vi "Test - All-In-One - SLAM Configuration -DISP B (SubVI).vi"(0 "START TEST":bool, 1 "STOP TEST":bool, 2 "NEXT STEP":bool, 3 "HOLD STEP":bool, 4 "Test Folder":path, 5 "Error Input":errorcluster, 7 "SLAM Test Cluster":T1={"Load Test"=0, "New Test Name"="", "Test Description"="", "Step Select"=0, "Save Test"=FALSE, "Erase Test"=FALSE, "Max Steps"=15, "Loop Limit"=5, "Continue at Loop Limit?"=FALSE, "Step N"=2, "Test Array (Standard)"=[{"Step Number"=0, "Step Description"="Turn ON H2O VLV", "Step Time Target"=1.0, "Step Time Unit"=0, "Step End Action"=0}, {"Step Number"=1, "Step Description"="H2O OFF, Soap ON", "Step Time Target"=1.0, "Step Time Unit"=0, "Step End Action"=0}, {"Step Number"=2, "Step Description"="Scrub Delay Time", "Step Time Target"=4.0, "Step Time Unit"=0, "Step End Action"=0}, {"Step Number"=3, "Step Description"="Rinse Time", "Step Time Target"=20.0, "Step Time Unit"=0, "Step End Action"=0}, {"Step Number"=4, "Step Description"="Signal Complete", "Step Time Target"=1.0, "Step Time Unit"=0, "Step End Action"=0}, {"Step Number"=5, "Step Description"="Re-Initialize", "Step Time Target"=0.5, "Step Time Unit"=0, "Step End Action"=3}], "Test Array (Custom)"=[{"Digital Outputs"=[TRUE, TRUE, FALSE, FALSE, FALSE, FALSE, FALSE, FALSE]}, {"Digital Outputs"=[FALSE, TRUE, TRUE, FALSE, FALSE, FALSE, FALSE, FALSE]}, {"Digital Outputs"=[FALSE, FALSE, FALSE, TRUE, FALSE, FALSE, FALSE, FALSE]}, {"Digital Outputs"=[TRUE, FALSE, FALSE, FALSE, TRUE, TRUE, FALSE, FALSE]}, {"Digital Outputs"=[FALSE, FALSE, FALSE, FALSE, FALSE, FALSE, TRUE, FALSE]}, {"Digital Outputs"=[FALSE, FALSE, FALSE, FALSE, FALSE, FALSE, FALSE, FALSE]}]} {"Test Array (Standard)"."Step End Action" items=["Go to Next Step", "Loop to Step 0", "Loop to Step N", "Stop Test Mode", "Stop Program"]; "Test Array (Standard)"."Step Time Unit" items=["sec", "min", "hr"]; "Test Array (Standard)"."Step Time Target" min=0.001 format="%#.3f"; "Test Array (Standard)"."Step Number" min=0 step=1; "Load Test" items=["123", "a", "b", "c"]; "Step Select" step=1}, 9 "SLAM Test Cluster Ref":refnum<vi>) -> (11 "Stop Program?":bool, 13 "Test Running?":bool, 14 "Test Display":string="Mode: OFF  (Press Start to Begin)\r\r\r    ", 15 "Test Output":cluster{"Digital Outputs":bool[]}, 16 "Step Complete?":bool=TRUE, 17 "Step Number":u16, 18 "Loop Number":u16, 19 "Error Output":errorcluster)   [LabVIEW 2012]
panel:
  # "Extra (Unused)"
  # "Red LED's"
  # "Rinse Green LED"
  # "+1 on Hand Remove"
  # "Scrub Green LED"
  # "Soap Control"
  # "Water Green LED"
  # "H2O Control"
  # "Scroll"
  # "Step"
  # "Description"
  # "Time Target"
  # "End Action"
  # "Total #\nof Steps"
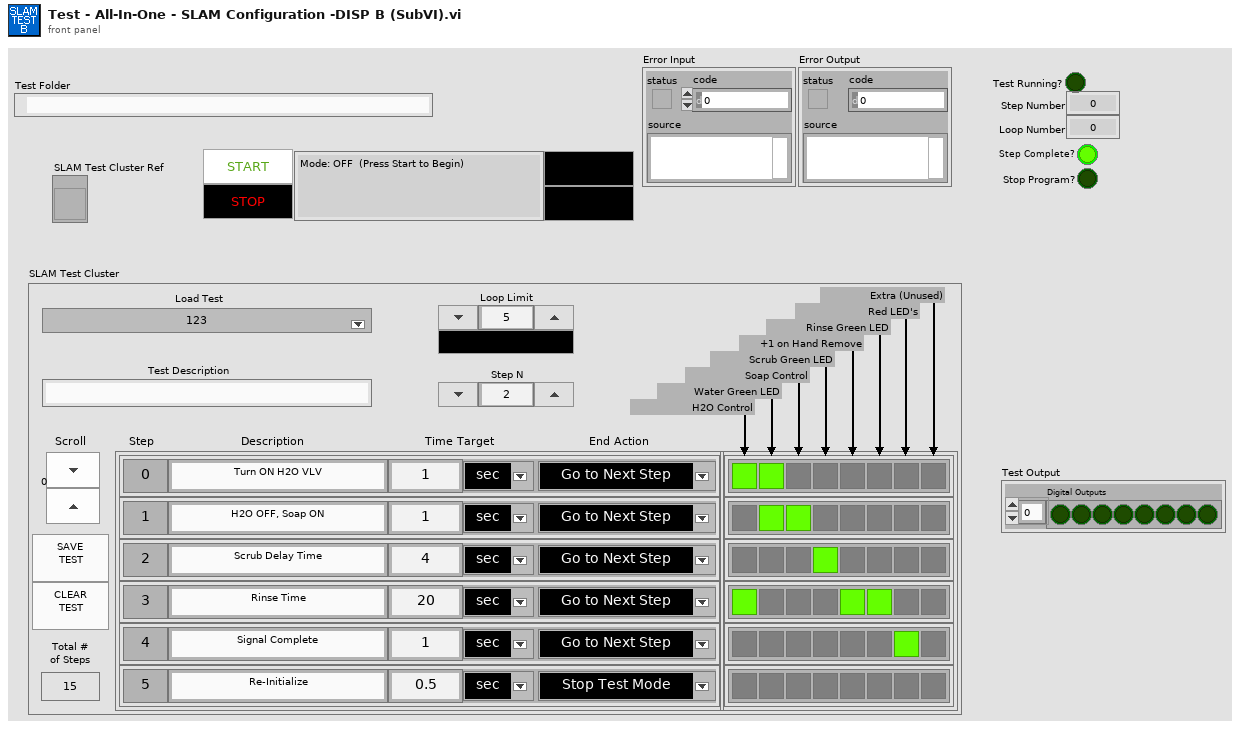
[diagram p1: front panel]
types:
  T1 = cluster{"Load Test":u16, "New Test Name":string, "Test Description":string, "Step Select":u16, "Save Test":bool, "Erase Test":bool, "Max Steps":u16, "Loop Limit":u16, "Continue at Loop Limit?":bool, "Step N":u16, "Test Array (Standard)":cluster{"Step Number":i32, "Step Description":string, "Step Time Target":dbl, "Step Time Unit":u16, "Step End Action":u16}[], "Test Array (Custom)":cluster{"Digital Outputs":bool[]}[]}
  T2 = cluster{"Load Test Ring":i32, "New Test Name":i32, "Test Description":i32, "Step Select":i32, "Save Test":i32, "Erase Test":i32, "Max Steps":i32, "Loop Limit":i32, "Continue at Loop Limit":i32, "Step N":i32, "Test Array (Standard)":i32, "Test Array (Custom)":i32}
  T3 = enum8{"Enabled", "Disabled", "Disabled and Grayed Out"}
  T4 = cluster{"Step Number":i32, "Step Description":string, "Step Time Target":dbl, "Step Time Unit":u16, "Step End Action":u16}[]
  T5 = enum16{"open", "replace", "create", "open or create", "replace or create", "replace or create with confirmation"}
  T6 = cluster{"Step Number":i32, "Step Description":string, "Step Time Target":dbl, "Step Time Unit":u16, "Step End Action":u16}
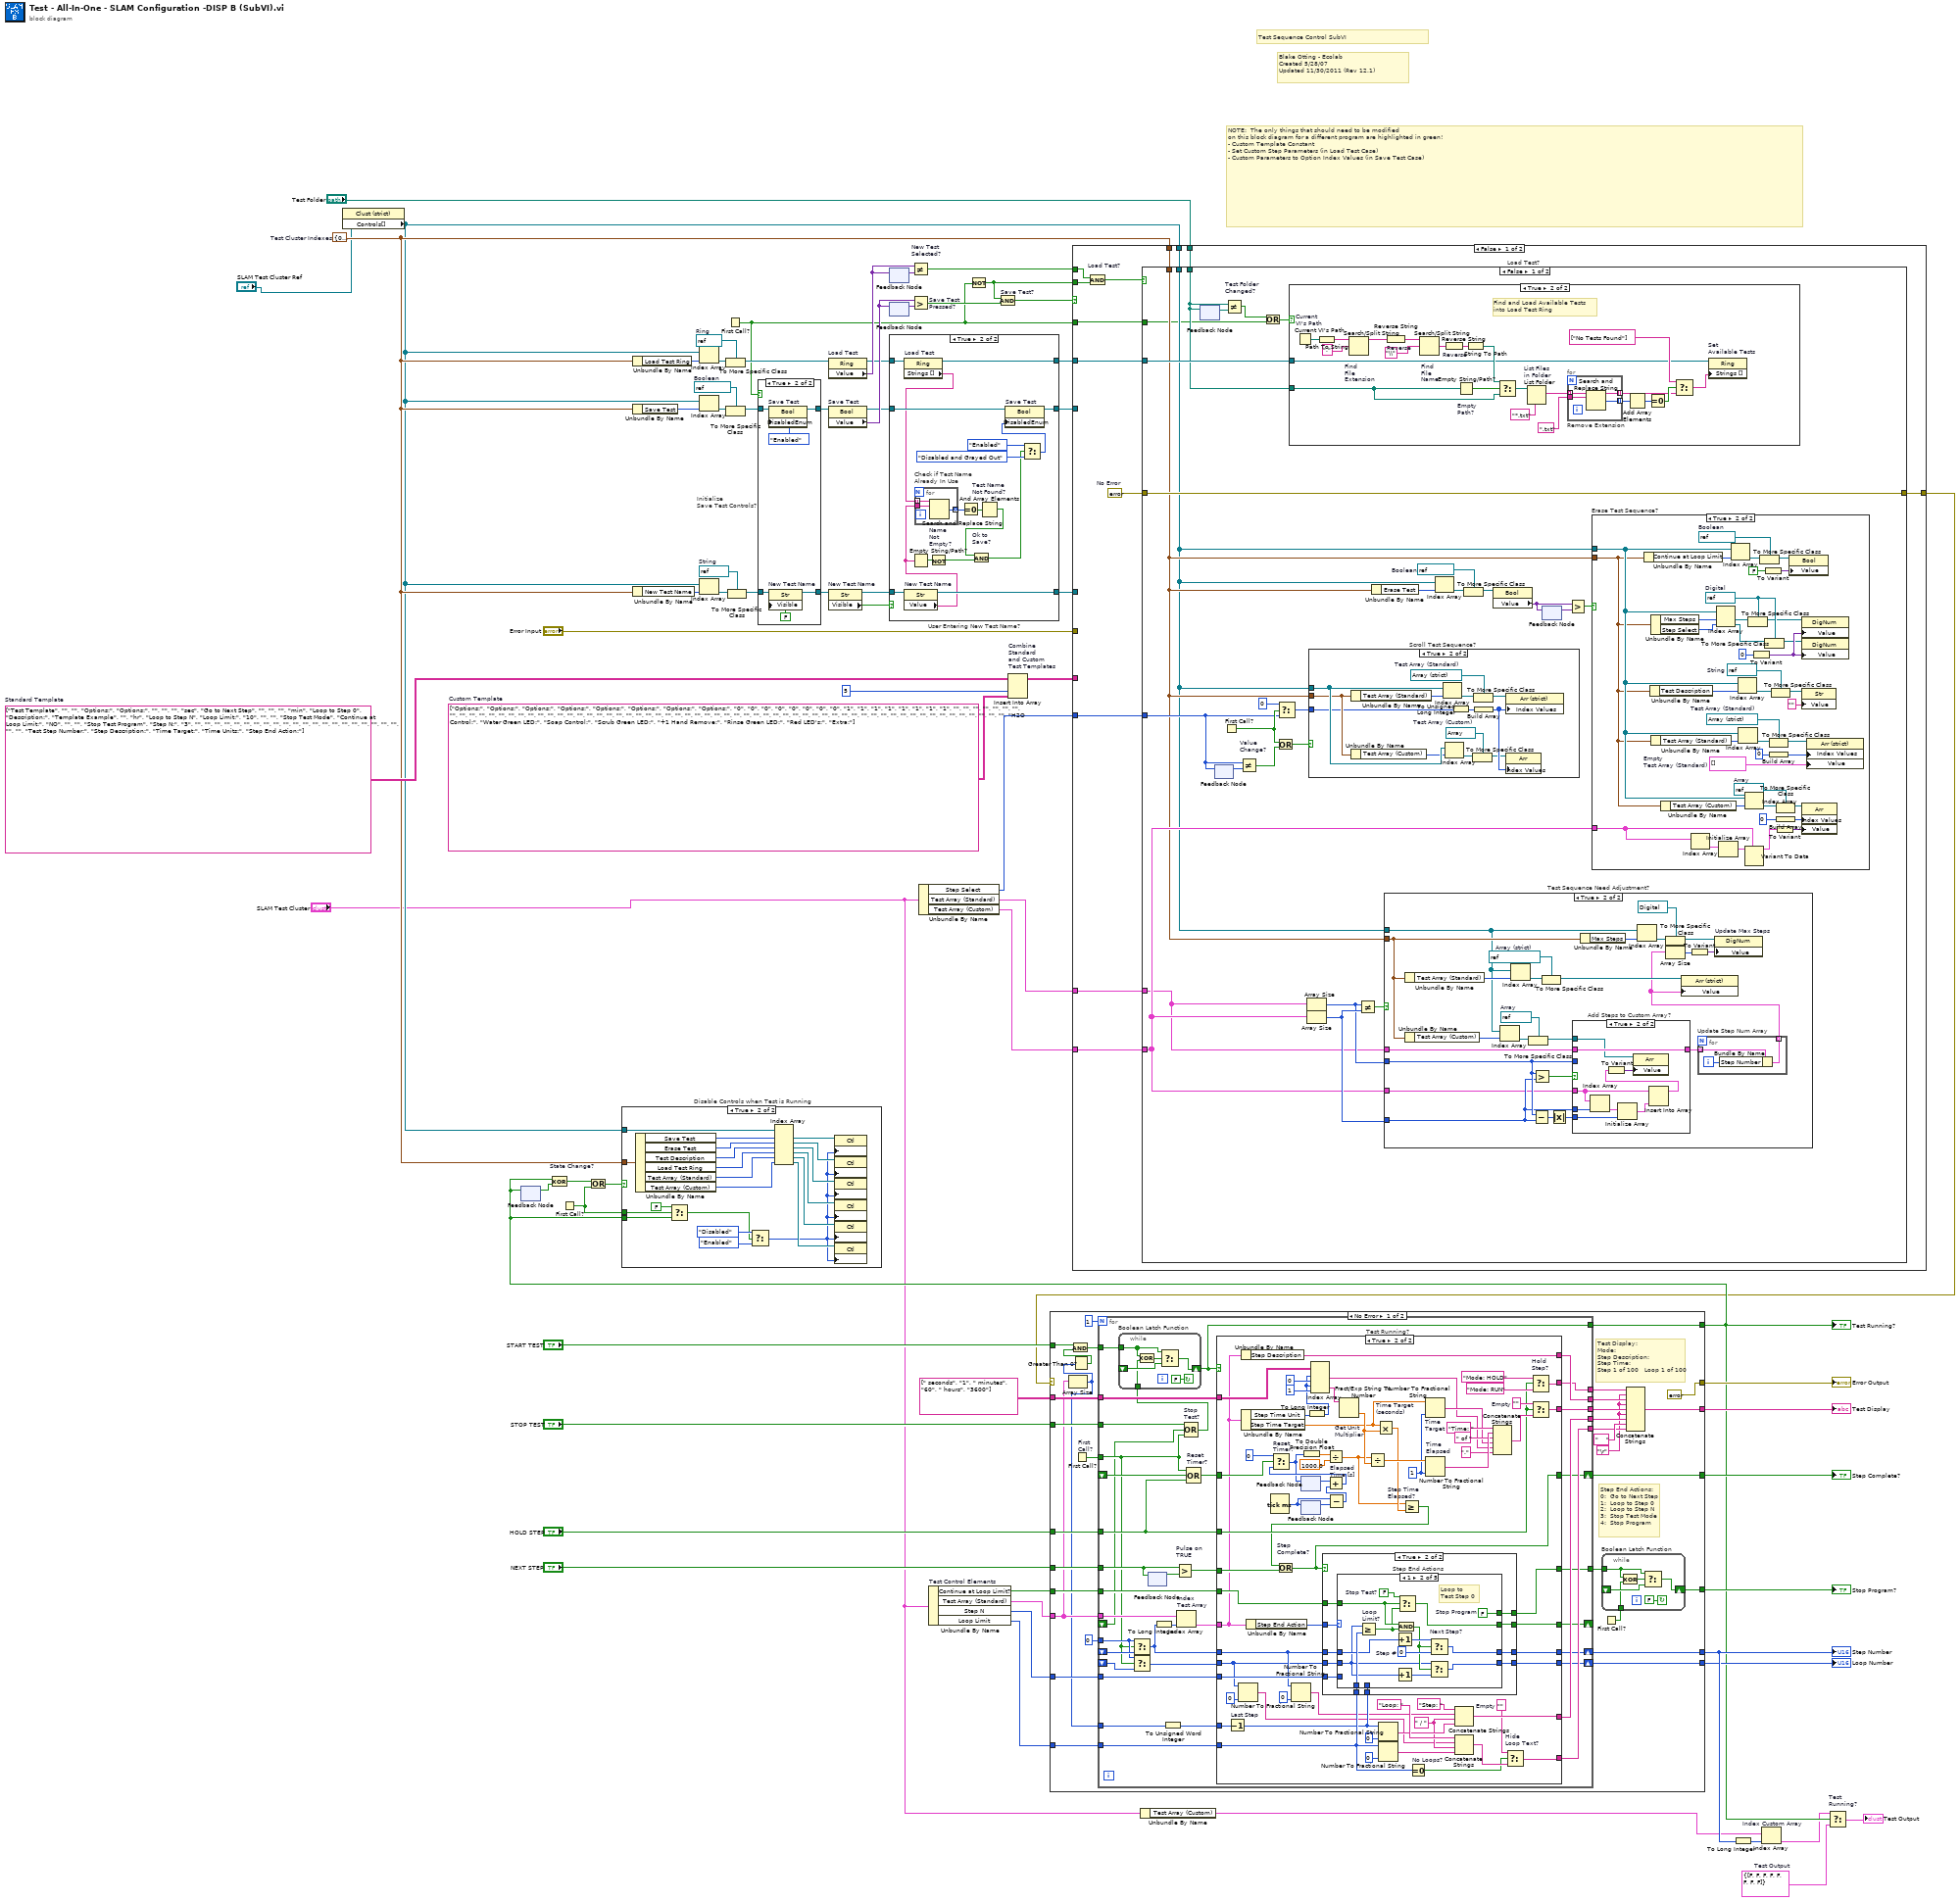
[diagram p0: block diagram]
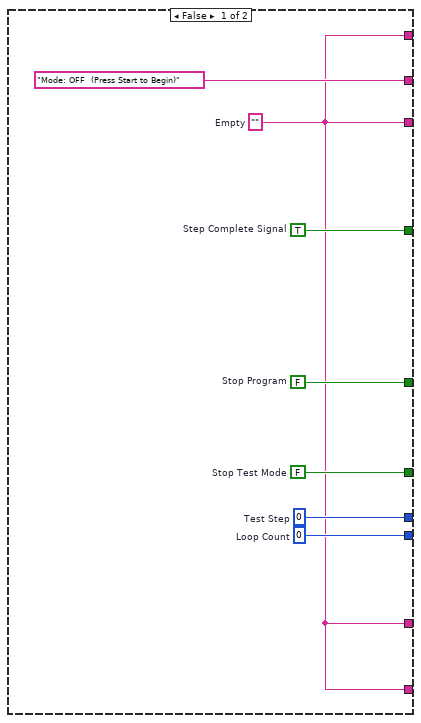
[diagram p3: hidden frame]
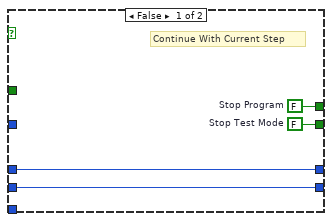
[diagram p4: hidden frame]
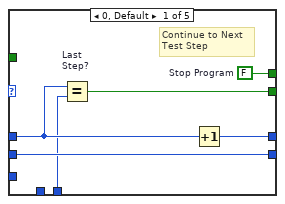
[diagram p5: hidden frame]
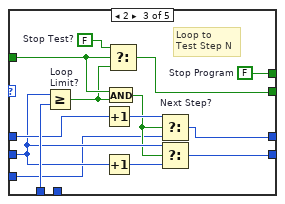
[diagram p6: hidden frame]
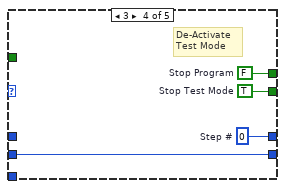
[diagram p7: hidden frame]
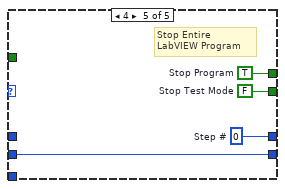
[diagram p8: hidden frame]
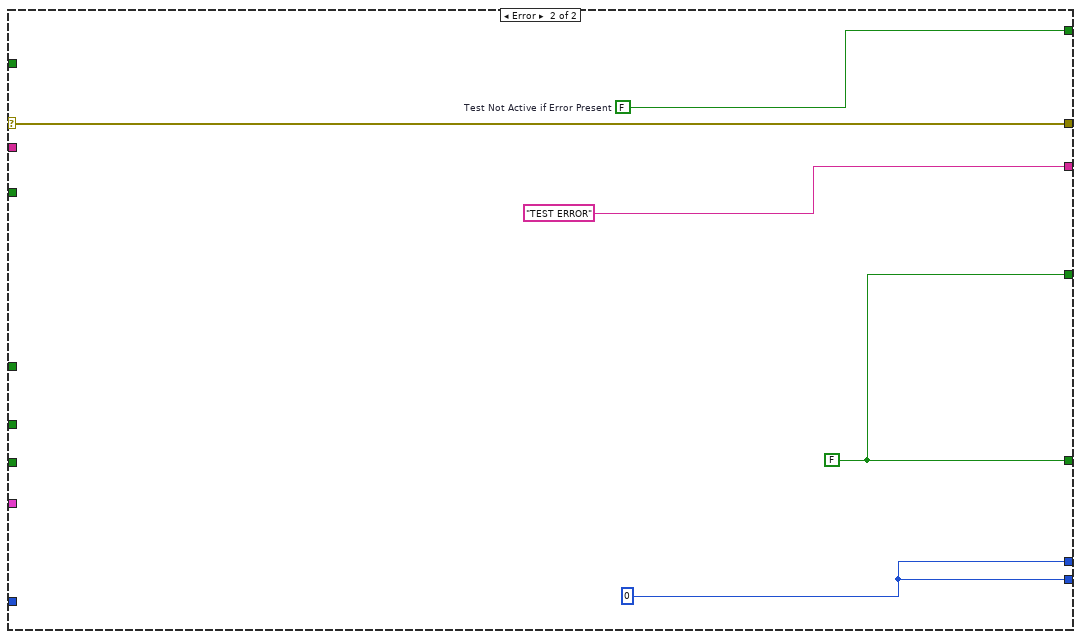
[diagram p9: hidden frame]
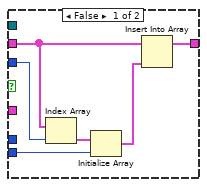
[diagram p13: hidden frame]
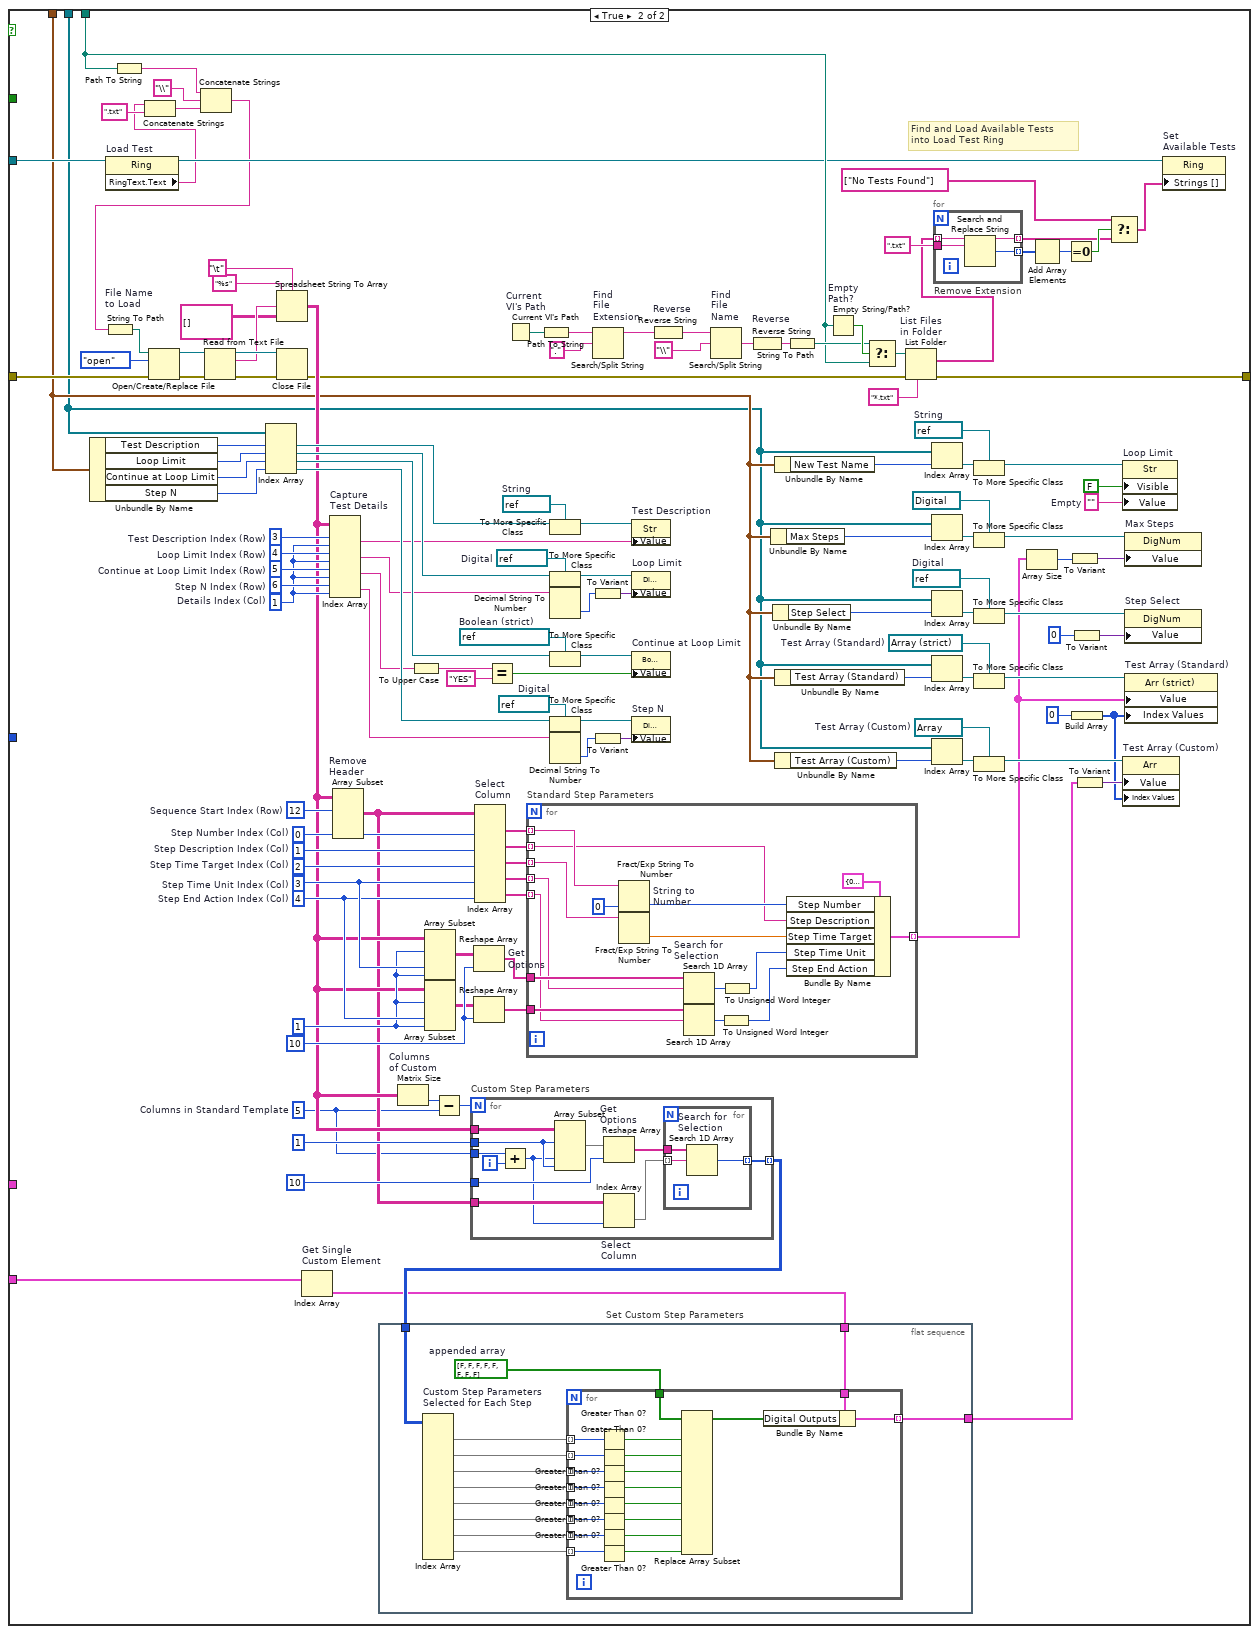
[diagram p17: hidden frame]
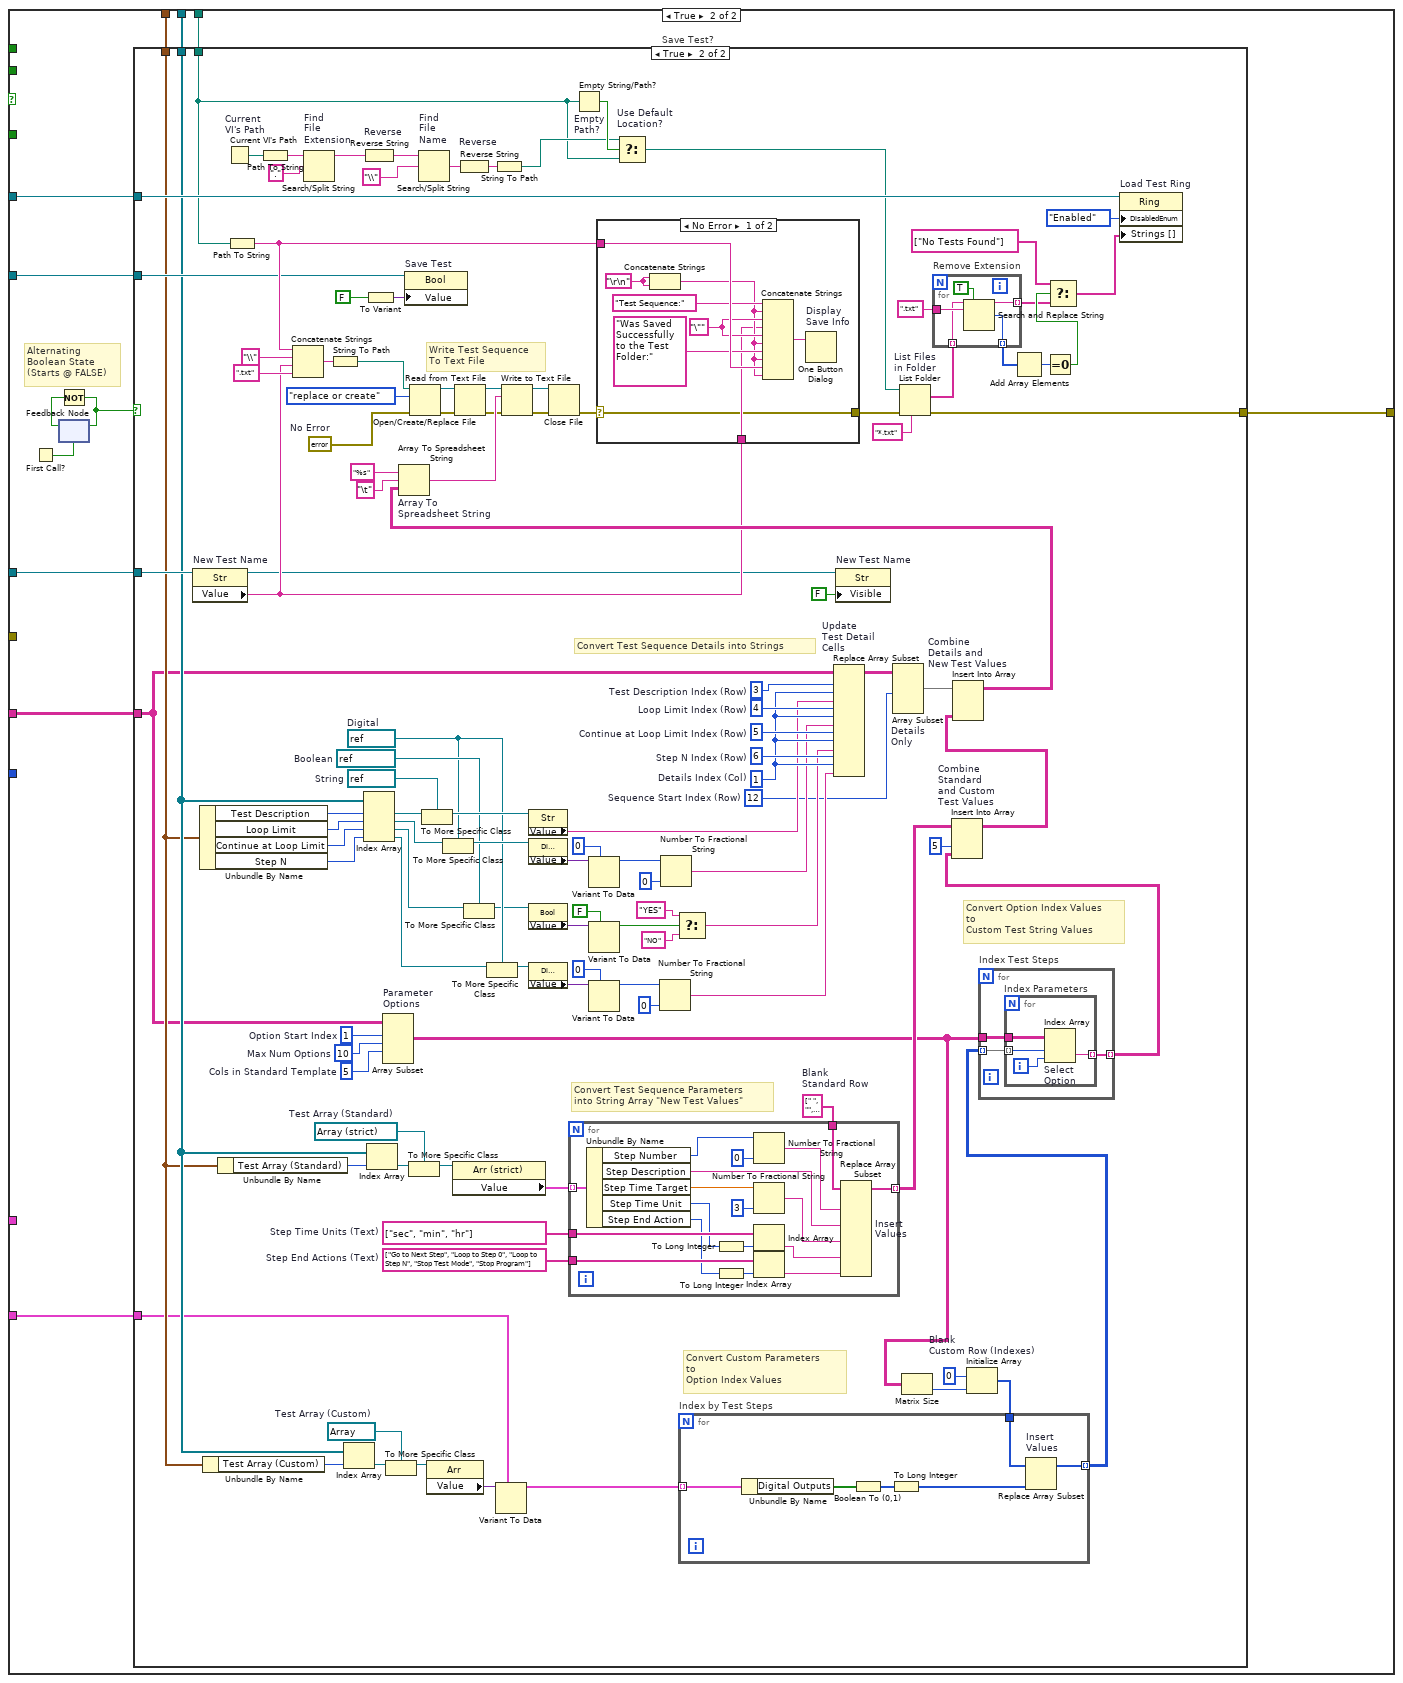
[diagram p18: hidden frame]
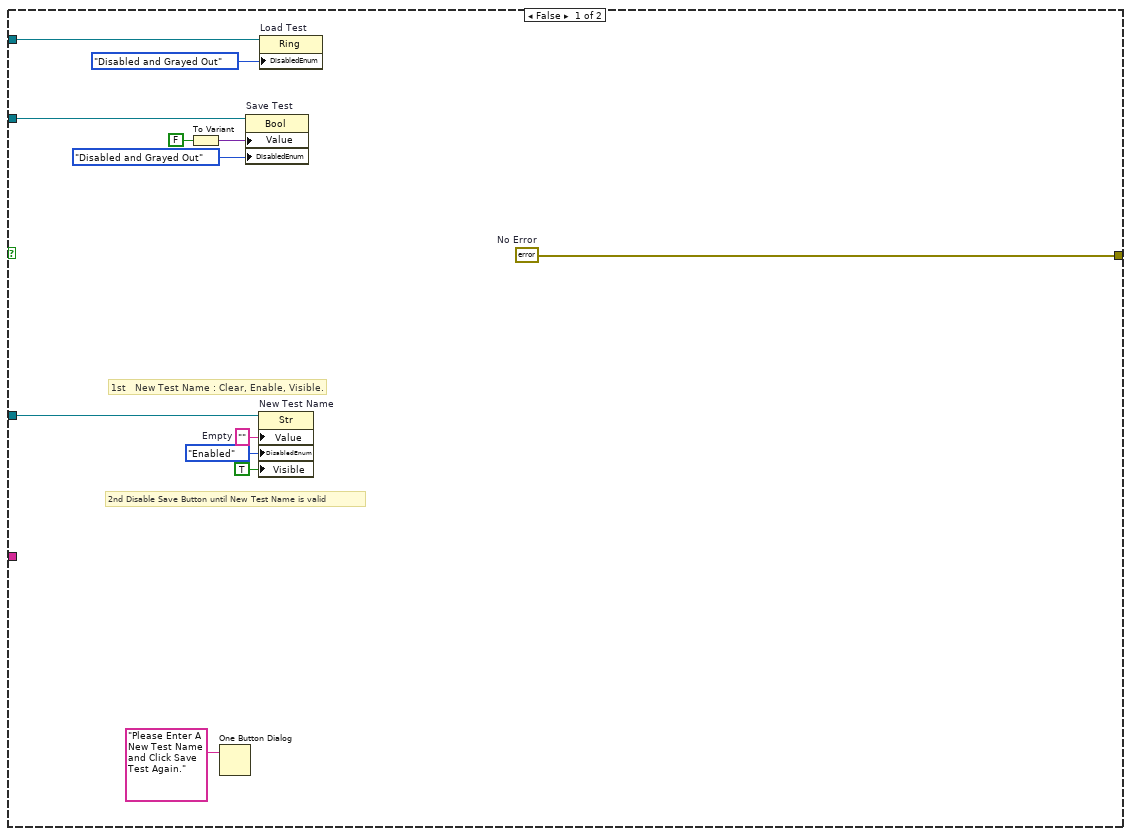
[diagram p19: hidden frame]
diagram:
  w2 = cluster{"Digital Outputs":bool[]} {"Digital Outputs"=[FALSE, FALSE, FALSE, FALSE, FALSE, FALSE, FALSE, FALSE]}  # Test Output
  w31 = refnum<vi> refnum  # Ring
  w53 = refnum<vi> refnum  # Boolean
  w57 = refnum<vi> refnum  # String
  w62 = string[][] [["Options:", "Options:", "Options:", "Options:", "Options:", "Options:", "Options:", "Options:"], ["0", "0", "0", "0", "0", "0", "0", "0"], ["1", "1", "1", "1", "1", "1", "1", "1"], ["", "", "", "", "", "", "", ""], ["", "", "", "", "", "", "", ""], ["", "", "", "", "", "", "", ""], ["", "", "", "", "", "", "", ""], ["", "", "", "", "", "", "", ""], ["", "", "", "", "", "", "", ""], ["", "", "", "", "", "", "", ""], ["", "", "", "", "", "", "", ""], ["H2O Control:", "Water Green LED:", "Soap Control:", "Scrub Green LED:", "+1 Hand Remove:", "Rinse Green LED:", "Red LED's:", "Extra:"]]  # Custom Template
  w64 = T2 {"Load Test Ring"=0, "New Test Name"=1, "Test Description"=2, "Step Select"=3, "Save Test"=4, "Erase Test"=5, "Max Steps"=6, "Loop Limit"=7, "Continue at Loop Limit"=8, "Step N"=9, "Test Array (Standard)"=10, "Test Array (Custom)"=11}  # Test Cluster Indexes
  w69 = string[][] [["Test Template", "", "", "Options:", "Options:"], ["", "", "", "sec", "Go to Next Step"], ["", "", "", "min", "Loop to Step 0"], ["Description:", "Template Example", "", "hr", "Loop to Step N"], ["Loop Limit:", "10", "", "", "Stop Test Mode"], ["Continue at Loop Limit:", "NO", "", "", "Stop Test Program"], ["Step N:", "3", "", "", ""], ["", "", "", "", ""], ["", "", "", "", ""], ["", "", "", "", ""], ["", "", "", "", ""], ["Test Step Number:", "Step Description:", "Time Target:", "Time Units:", "Step End Action:"]]  # Standard Template
  # "NOTE:  The only things that should need to be modified\non this block diagram for a different program are highlighted in green!\n- Custom Template Constant\n- Set Custom Step Parameters (in Load Test Case)\n- Custom Parameters to Option Index Values (in Save Test Case)"
  # "Blake Otting - Ecolab\nCreated 5/28/07\nUpdated 11/30/2011 (Rev 12.1)"
  # "Test Sequence Control SubVI"
  n1 = property class="Clust (strict)"(reference="SLAM Test Cluster Ref") -> ("Controls[]"=w63:refnum<vi>[])  [unwired: 1 in, 2 out]
  n2 = feedback #1() -> (w28:bool)  [unwired: 1 in]
  n3 = First Call?() -> (First Call?: T/F=w25:bool)
  n4 = Unbundle By Name(w64) -> ("Load Test Ring"=w32:i32)
  n5 = Unbundle By Name(w64) -> ("Save Test"=w55:i32)
  n6 = Unbundle By Name(w64) -> ("New Test Name"=w59:i32)
  n7 = Index Array(array=w63, index=w32) -> (element=w30:refnum<vi>)
  n8 = Index Array(array=w63, index=w55) -> (element=w54:refnum<vi>)
  n9 = Index Array(array=w63, index=w59) -> (element=w58:refnum<vi>)
  n10 = First Call?() -> (First Call?: T/F=w11:bool)
  n11 = To More Specific Class(target class=w31, reference=w30) -> (specific class reference=w29:refnum<vi>)  [unwired: 1 in, 1 out]
  n12 = To More Specific Class(target class=w53, reference=w54) -> (specific class reference=w42:refnum<vi>)  [unwired: 1 in, 1 out]
  n13 = To More Specific Class(target class=w57, reference=w58) -> (specific class reference=w44:refnum<vi>)  [unwired: 1 in, 1 out]
  n14 = case "Initialize\nSave Test Controls?" shown="True" w11 {
    tunnel: w42 -> [w70 w77]
    tunnel: [w70 w76] -> w41
    tunnel: w44 -> [w71 w75]
    tunnel: [w71 w74] -> w43
    frame False {
    }
    frame True {
      n15 = property on="Save Test" class="Bool"(reference=w77, "DisabledEnum"=T3."Enabled" ("Disabled")) -> (reference out=w76:refnum<vi>)  [unwired: 1 in, 1 out]
      n16 = property on="New Test Name" class="Str"(reference=w75, "Visible"=FALSE) -> (reference out=w74:refnum<vi>)  [unwired: 1 in, 1 out]
    }
  }
  n17 = property on="Load Test" class="Ring"(reference=w29) -> (reference out=w37:refnum<vi>, "Value"=w38:variant)  [unwired: 1 in, 1 out]
  n18 = property on="Save Test" class="Bool"(reference=w41) -> (reference out=w47:refnum<vi>, "Value"=w51:variant)  [unwired: 1 in, 1 out]
  n19 = property on="New Test Name" class="Str"(reference=w43) -> (reference out=w49:refnum<vi>, "Visible"=w50:bool)  [unwired: 1 in, 1 out]
  n20 = case "User Entering New Test Name?" shown="True" w50 {
    tunnel: w49 -> [w80 w93]
    tunnel: w37 -> [w79 w92]
    tunnel: [w80 w88] -> w46
    tunnel: [w79 w87] -> w48
    tunnel: w47 -> [w78 w86]
    tunnel: [w78 w85] -> w45
    frame False {
    }
    frame True {
      n21 = property on="Load Test" class="Ring"(reference=w92) -> (reference out=w87:refnum<vi>, "Strings []"=w82:string[])  [unwired: 1 in, 1 out]
      n22 = property on="New Test Name" class="Str"(reference=w93) -> (reference out=w88:refnum<vi>, "Value"=w81:string)  [unwired: 1 in, 1 out]
      n23 = Empty String/Path?(string/path=w81) -> (empty?=w94:bool)
      n24 = for "Check if Test Name\nAlready In Use" {
        tunnel: w82 -> [w100] mode=indexing
        tunnel: w81 -> [w99]
        tunnel: [w98] -> w97 mode=indexing
        n25 = Search and Replace String(input string=w100, search string=w99) -> (number of replacements=w98:i32)  [unwired: 6 in, 3 out]
      }
      n26 = Not "Name\nNot\nEmpty?"(x=w94) -> (.not. x?=w89:bool)
      n27 = Equal To 0?(x=w97) -> (x = 0?=w96:bool[])
      n28 = And Array Elements "Test Name\nNot Found?"(Boolean array=w96) -> (logical AND=w95:bool)
      n29 = And "Ok to\nSave?"(x=w95, y=w89) -> (x .and. y?=w83:bool)
      n30 = Select(t=T3."Enabled" ("Disabled"), s=w83, f=T3."Disabled and Grayed Out" ("Disabled")) -> (s? t:f=w84:T3)
      n31 = property on="Save Test" class="Bool"(reference=w86, "DisabledEnum"=w84) -> (reference out=w85:refnum<vi>)  [unwired: 1 in, 1 out]
    }
  }
  n32 = feedback #2() -> (w39:variant)  [unwired: 1 in]
  n33 = feedback-in #2(w38) -> ()
  n34 = feedback #3() -> (w52:variant)  [unwired: 1 in]
  n35 = feedback-in #3(w51) -> ()
  n36 = Not Equal? "New Test\nSelected?"(x=w38, y=w39) -> (x != y?=w7:bool)
  n37 = Greater? "Save Test\nPressed?"(x=w51, y=w52) -> (0:w36:bool)
  n38 = Unbundle By Name("SLAM Test Cluster") -> ("Step Select"=w19:u16, "Test Array (Standard)"=w21:T4, "Test Array (Custom)"=w20:cluster{"Digital Outputs":bool[]}[])
  n39 = Unbundle By Name "Test Control Elements"("SLAM Test Cluster") -> ("Continue at Loop Limit?"=w24:bool, "Test Array (Standard)"=w9:T4, "Step N"=w23:u16, "Loop Limit"=w22:u16)
  n40 = Not(x=w11) -> (.not. x?=w35:bool)
  n41 = And "Save Test?"(x=w35, y=w36) -> (x .and. y?=w40:bool)
  n42 = Insert Into Array "Combine\nStandard\nand Custom\nTest Templates"(array=w69, index (col)=5 ("disabled index (col)"), new element=w62) -> (w56:string[][])  [unwired: 1 in]
  n43 = case shown="False" w40 {
    tunnel: "Test Folder" -> [w109 w465]
    tunnel: w20 -> [w110 w466]
    tunnel: w56 -> [_ w467]
    tunnel: w64 -> [w112 w471]
    tunnel: w63 -> [w113 w472]
    tunnel: w45 -> [_ w470]
    tunnel: w46 -> [_ w469]
    tunnel: w48 -> [w111 w468]
    tunnel: [w104 w464] -> w10
    tunnel: "Error Input" -> [_ _]
    tunnel: w7 -> [w106 _]
    tunnel: w11 -> [w108 _]
    tunnel: w35 -> [w105 _]
    tunnel: w19 -> [w103 _]
    tunnel: w21 -> [w102 _]
    frame False {
      w101 = errorcluster {"status"=FALSE, "code"=0, "source"=""}  # No Error
      n44 = And "Load Test?"(x=w106, y=w105) -> (x .and. y?=w107:bool)
      n45 = case "Load Test?" shown="False" w107 {
        tunnel: w113 -> [w120 w265]
        tunnel: w112 -> [w121 w266]
        tunnel: w110 -> [w122 w397]
        tunnel: [w141 w274] -> w104
        tunnel: w101 -> [w141 w267]
        tunnel: w111 -> [w140 w271]
        tunnel: w108 -> [w115 _]
        tunnel: w109 -> [w117 w272]
        tunnel: w103 -> [w133 _]
        tunnel: w102 -> [w119 _]
        frame False {
          w128 = refnum<vi> refnum  # Boolean
          n46 = feedback #4() -> (w118:path)  [unwired: 1 in]
          n47 = feedback-in #4(w117) -> ()
          n48 = feedback #5() -> (w134:u16)  [unwired: 1 in]
          n49 = feedback-in #5(w133) -> ()
          n50 = First Call?() -> (First Call?: T/F=w138:bool)
          n51 = Not Equal? "Test Folder\nChanged?"(x=w117, y=w118) -> (x != y?=w116:bool)
          n52 = Not Equal? "Value\nChange?"(x=w133, y=w134) -> (x != y?=w135:bool)
          n53 = Or(x=w116, y=w115) -> (x .or. y?=w114:bool)
          n54 = Or(x=w138, y=w135) -> (x .or. y?=w136:bool)
          n55 = Select(t=u16 0 ("upper limit"), s=w138, f=w133) -> (s? t:f=w139:u16)
          n56 = case shown="True" w114 {
            tunnel: w140 -> [_ w239]
            tunnel: w117 -> [_ w238]
            frame False {
            }
            frame True {
              # "Find and Load Available Tests \ninto Load Test Ring"
              n57 = Current VI's Path "Current\nVI's Path"() -> (path=w249:path)
              n58 = Path To String(path=w249) -> (string=w254:string)
              n59 = Search/Split String "Find\nFile \nExtension"(string=w254, search string/char (-)=".") -> (substring before match=w253:string)  [unwired: 1 in, 2 out]
              n60 = Reverse String "Reverse"(1:w253) -> (0:w252:string)
              n61 = Search/Split String "Find\nFile \nName"(string=w252, search string/char (-)="\\") -> (match + rest of string=w250:string)  [unwired: 1 in, 2 out]
              n62 = Reverse String "Reverse"(1:w250) -> (0:w256:string)
              n63 = Empty String/Path? "Empty\nPath?"(string/path=w238) -> (empty?=w248:bool)
              n64 = String To Path(string=w256) -> (path=w247:path)
              n65 = Select(t=w247, s=w248, f=w238) -> (s? t:f=w257:path)
              n66 = List Folder "List Files\nin Folder"(path=w257, pattern="*.txt") -> (filenames=w259:string[])  [unwired: 1 in, 4 out]
              n67 = for "Remove Extension" {
                tunnel: w259 -> [w262] mode=indexing
                tunnel: ".txt" ("pattern") -> [w263]
                tunnel: [w261] -> w240 mode=indexing
                tunnel: [w260] -> w245 mode=indexing
                n68 = Search and Replace String(input string=w262, search string=w263) -> (result string=w261:string, number of replacements=w260:i32)  [unwired: 6 in, 2 out]
              }
              n69 = Add Array Elements(numeric array=w245) -> (sum=w244:i32)
              n70 = Equal To 0?(x=w244) -> (x = 0?=w243:bool)
              n71 = Select(t=string[] ["No Tests Found"], s=w243, f=w240) -> (s? t:f=w242:string[])
              n72 = property on="Set\nAvailable Tests" class="Ring"(reference=w239, "Strings []"=w242) -> ()  [unwired: 1 in, 2 out]
            }
          }
          n73 = Array Size(array=w119) -> (size(s)=w123:i32)
          n74 = Array Size(array=w122) -> (size(s)=w124:i32)
          n75 = case "Scroll Test Sequence?" shown="True" w136 {
            tunnel: w120 -> [_ w237]
            tunnel: w121 -> [_ w236]
            tunnel: w139 -> [_ w225]
            frame False {
            }
            frame True {
              w235 = refnum<vi> refnum  # Test Array (Custom)
              w232 = refnum<vi> refnum  # Test Array (Standard)
              n76 = Unbundle By Name(w236) -> ("Test Array (Standard)"=w233:i32)
              n77 = Unbundle By Name(w236) -> ("Test Array (Custom)"=w234:i32)
              n78 = Index Array(array=w237, index=w233) -> (element=w226:refnum<vi>)
              n79 = Index Array(array=w237, index=w234) -> (element=w229:refnum<vi>)
              n80 = To Unsigned Long Integer(number=w225) -> (unsigned 32bit integer=w228:u32)
              n81 = To More Specific Class(target class=w235, reference=w229) -> (specific class reference=w230:refnum<vi>)  [unwired: 1 in, 1 out]
              n82 = To More Specific Class(target class=w232, reference=w226) -> (specific class reference=w227:refnum<vi>)  [unwired: 1 in, 1 out]
              n83 = Build Array(w228) -> (w231:u32[])
              n84 = property class="Arr (strict)"(reference=w227, "Index Values"=w231) -> ()  [unwired: 1 in, 2 out]
              n85 = property class="Arr"(reference=w230, "Index Values"=w231) -> ()  [unwired: 1 in, 2 out]
            }
          }
          n86 = Not Equal?(x=w123, y=w124) -> (x != y?=w125:bool)
          n87 = Unbundle By Name(w121) -> ("Erase Test"=w126:i32)
          n88 = case "Test Sequence Need Adjustment?" shown="True" w125 {
            tunnel: w121 -> [_ w150]
            tunnel: w120 -> [_ w149]
            tunnel: w123 -> [_ w148]
            tunnel: w119 -> [_ w147]
            tunnel: w124 -> [_ w146]
            tunnel: w122 -> [_ w145]
            frame False {
            }
            frame True {
              w162 = refnum<vi> refnum  # Array
              w159 = refnum<vi> refnum  # Array (strict)
              n89 = Unbundle By Name(w150) -> ("Test Array (Standard)"=w160:i32)
              n90 = Unbundle By Name(w150) -> ("Test Array (Custom)"=w161:i32)
              n91 = Index Array(array=w149, index=w161) -> (element=w158:refnum<vi>)
              n92 = Index Array(array=w149, index=w160) -> (element=w157:refnum<vi>)
              n93 = To More Specific Class(target class=w162, reference=w158) -> (specific class reference=w144:refnum<vi>)  [unwired: 1 in, 1 out]
              n94 = Subtract(x=w148, y=w146) -> (x-y=w165:i32)
              n95 = Greater?(x=w148, y=w146) -> (0:w164:bool)
              n96 = To More Specific Class(target class=w159, reference=w157) -> (specific class reference=w143:refnum<vi>)  [unwired: 1 in, 1 out]
              n97 = Absolute Value(x=w165) -> (abs(x)=w166:i32)
              n98 = case "Add Steps to Custom Array?" shown="True" w164 {
                tunnel: w144 -> [_ w173]
                tunnel: w146 -> [_ w174]
                tunnel: w145 -> [_ w180]
                tunnel: w147 -> [w168 w175]
                tunnel: w166 -> [w172 w176]
                tunnel: w148 -> [w171 _]
                tunnel: [w167 w175] -> w163
                frame False {
                  n99 = Index Array(array=w168, index=w171) -> (element=w170:T6)
                  n100 = Initialize Array(w170, w172) -> (w169:T4)
                  n101 = Insert Into Array(array=w168, new element=w169) -> (w167:T4)  [unwired: 1 in]
                }
                frame True {
                  n102 = Index Array(array=w180, index=w174) -> (element=w181:cluster{"Digital Outputs":bool[]})
                  n103 = Initialize Array(w181, w176) -> (w179:cluster{"Digital Outputs":bool[]}[])
                  n104 = Insert Into Array(array=w180, new element=w179) -> (w178:cluster{"Digital Outputs":bool[]}[])  [unwired: 1 in]
                  n105 = To Variant(anything=w178) -> (Variant=w177:variant)
                  n106 = property class="Arr"(reference=w173, "Value"=w177) -> ()  [unwired: 1 in, 2 out]
                }
              }
              n107 = Unbundle By Name(w150) -> ("Max Steps"=w156:i32)
              n108 = Index Array(array=w149, index=w156) -> (element=w152:refnum<vi>)
              n109 = To More Specific Class(target class=refnum<vi> refnum ("Max Steps"), reference=w152) -> (specific class reference=w155:refnum<vi>)  [unwired: 1 in, 1 out]
              n110 = for "Update Step Num Array" {
                tunnel: w163 -> [w184] mode=indexing
                tunnel: [w182] -> w142 mode=indexing
                i -> [w183]
                n111 = Bundle By Name(cluster=w184, "Step Number"=w183) -> (w182:T6)
              }
              n112 = Array Size(array=w142) -> (size(s)=w151:i32)
              n113 = property class="Arr (strict)"(reference=w143, "Value"=w142) -> ()  [unwired: 1 in, 2 out]
              n114 = To Variant(anything=w151) -> (Variant=w153:variant)
              n115 = property on="Update Max Steps" class="DigNum"(reference=w155, "Value"=w153) -> ()  [unwired: 1 in, 2 out]
            }
          }
          n116 = Index Array(array=w120, index=w126) -> (element=w127:refnum<vi>)
          n117 = To More Specific Class(target class=w128, reference=w127) -> (specific class reference=w129:refnum<vi>)  [unwired: 1 in, 1 out]
          n118 = property class="Bool"(reference=w129) -> ("Value"=w130:variant)  [unwired: 1 in, 2 out]
          n119 = feedback #6() -> (w131:variant)  [unwired: 1 in]
          n120 = feedback-in #6(w130) -> ()
          n121 = Greater?(x=w130, y=w131) -> (0:w132:bool)
          n122 = case "Erase Test Sequence?" shown="True" w132 {
            tunnel: w122 -> [_ w207]
            tunnel: w121 -> [_ w190]
            tunnel: w120 -> [_ w191]
            frame False {
            }
            frame True {
              w188 = refnum<vi> refnum  # Boolean
              w221 = refnum<vi> refnum  # Digital
              w214 = refnum<vi> refnum  # String
              w205 = refnum<vi> refnum  # Array
              w198 = T4 []  # Empty Test Array (Standard)
              w197 = refnum<vi> refnum  # Test Array (Standard)
              n123 = Unbundle By Name(w190) -> ("Continue at Loop Limit"=w189:i32)
              n124 = Unbundle By Name(w190) -> ("Test Description"=w212:i32)
              n125 = Unbundle By Name(w190) -> ("Max Steps"=w224:i32, "Step Select"=w219:i32)
              n126 = Unbundle By Name(w190) -> ("Test Array (Standard)"=w203:i32)
              n127 = Unbundle By Name(w190) -> ("Test Array (Custom)"=w204:i32)
              n128 = Index Array(array=w207) -> (element=w206:cluster{"Digital Outputs":bool[]})  [unwired: 1 in]
              n129 = Index Array(array=w191, index #1=w224, index #2=w219) -> (element #1=w217:refnum<vi>, element #2=w220:refnum<vi>)
              n130 = Initialize Array(w206) -> (w210:cluster{"Digital Outputs":bool[]}[])  [unwired: 1 in]
              n131 = Index Array(array=w191, index=w189) -> (element=w192:refnum<vi>)
              n132 = Index Array(array=w191, index=w212) -> (element=w213:refnum<vi>)
              n133 = Index Array(array=w191, index=w203) -> (element=w193:refnum<vi>)
              n134 = Index Array(array=w191, index=w204) -> (element=w199:refnum<vi>)
              n135 = Variant To Data(type=w207, Variant=w210) -> (data=w208:cluster{"Digital Outputs":bool[]}[])  [unwired: 1 in, 1 out]
              n136 = To More Specific Class(target class=w221, reference=w217) -> (specific class reference=w218:refnum<vi>)  [unwired: 1 in, 1 out]
              n137 = To Variant(anything=0 ("Value")) -> (Variant=w223:variant)
              n138 = To More Specific Class(target class=w188, reference=w192) -> (specific class reference=w185:refnum<vi>)  [unwired: 1 in, 1 out]
              n139 = To Variant(anything=FALSE) -> (Variant=w187:variant)
              n140 = To More Specific Class(target class=w221, reference=w220) -> (specific class reference=w222:refnum<vi>)  [unwired: 1 in, 1 out]
              n141 = To More Specific Class(target class=w197, reference=w193) -> (specific class reference=w194:refnum<vi>)  [unwired: 1 in, 1 out]
              n142 = Build Array(u32 0 ("unsigned 32bit integer")) -> (w195:u32[])
              n143 = To More Specific Class(target class=w214, reference=w213) -> (specific class reference=w215:refnum<vi>)  [unwired: 1 in, 1 out]
              n144 = To Variant(anything=w208) -> (Variant=w209:variant)
              n145 = To More Specific Class(target class=w205, reference=w199) -> (specific class reference=w200:refnum<vi>)  [unwired: 1 in, 1 out]
              n146 = Build Array(u32 0 ("unsigned 32bit integer")) -> (w202:u32[])
              n147 = property class="Bool"(reference=w185, "Value"=w187) -> ()  [unwired: 1 in, 2 out]
              n148 = property class="DigNum"(reference=w218, "Value"=w223) -> ()  [unwired: 1 in, 2 out]
              n149 = property class="DigNum"(reference=w222, "Value"=w223) -> ()  [unwired: 1 in, 2 out]
              n150 = property class="Str"(reference=w215, "Value"="") -> ()  [unwired: 1 in, 2 out]
              n151 = property class="Arr"(reference=w200, "Index Values"=w202, "Value"=w209) -> ()  [unwired: 1 in, 2 out]
              n152 = property class="Arr (strict)"(reference=w194, "Index Values"=w195, "Value"=w198) -> ()  [unwired: 1 in, 2 out]
            }
          }
        }
        frame True {
          w298 = ""  # Empty
          w302 = refnum<vi> refnum  # String
          w307 = refnum<vi> refnum  # Digital
          w312 = refnum<vi> refnum  # Test Array (Custom)
          w320 = 5  # Columns in Standard Template
          w394 = 2  # Step Time Target Index (Col)
          w395 = 1  # Step Description Index (Col)
          w396 = 0  # Step Number Index (Col)
          w375 = refnum<vi> refnum  # Test Array (Standard)
          w372 = refnum<vi> refnum  # Digital
          w368 = refnum<vi> refnum  # Boolean (strict)
          w367 = refnum<vi> refnum  # Digital
          w353 = refnum<vi> refnum  # String
          w361 = 6  # Step N Index (Row)
          w360 = 5  # Continue at Loop Limit Index (Row)
          w359 = 4  # Loop Limit Index (Row)
          w358 = 3  # Test Description Index (Row)
          w336 = 1  # Details Index (Col)
          w392 = 4  # Step End Action Index (Col)
          w346 = 10 ("dimension size")
          w347 = 1 ("index")
          w393 = 3  # Step Time Unit Index (Col)
          w337 = 12  # Sequence Start Index (Row)
          # "Find and Load Available Tests \ninto Load Test Ring"
          n153 = Unbundle By Name(w266) -> ("Test Description"=w357:i32, "Loop Limit"=w354:i32, "Continue at Loop Limit"=w355:i32, "Step N"=w356:i32)
          n154 = property on="Load Test" class="Ring"(reference=w271) -> (reference out=w270:refnum<vi>, "RingText.Text"=w269:string)  [unwired: 1 in, 1 out]
          n155 = Path To String(path=w272) -> (string=w379:string)
          n156 = Concatenate Strings(w269, ".txt" ("string")) -> (w381:string)
          n157 = Concatenate Strings(w379, "\\" ("string"), w381) -> (w268:string)
          n158 = String To Path "File Name\nto Load"(string=w268) -> (path=w388:path)
          n159 = Open/Create/Replace File(file path (use dialog)=w388, error in=w267, operation (0:open)=T5."open") -> (refnum out=w390:refnum<file>, error out=w383:errorcluster)  [unwired: 3 in, 1 out]
          n160 = Read from Text File(file (use dialog)=w390, error in=w383) -> (refnum out=w391:refnum<file>, text=w389:string, error out=w382:errorcluster)  [unwired: 3 out]
          n161 = Index Array(array=w265, index #1=w357, index #2=w354, index #3=w355, index #4=w356) -> (element #1=w362:refnum<vi>, element #2=w363:refnum<vi>, element #3=w364:refnum<vi>, element #4=w365:refnum<vi>)
          n162 = Spreadsheet String To Array(delimiter (Tab)="\t" ("delimiter (\\t)"), format string="%s" ("format (%s)"), spreadsheet string=w389, array type (2D Dbl)=string[][] [] ("appended array")) -> (array=w323:string[][])
          n163 = Close File(refnum=w391, error in=w382) -> (error out=w275:errorcluster)  [unwired: 1 out]
          n164 = Index Array "Get Single\nCustom Element"(array=w397) -> (element=w318:cluster{"Digital Outputs":bool[]})  [unwired: 1 in]
          n165 = Index Array "Capture\nTest Details"(array=w323, index (row) #1=w358, index (col) #1=w336, index (row) #2=w359, index (col) #2=w336, index (row) #3=w360, index (col) #3=w336, index (row) #4=w361, index (col) #4=w336) -> (element #1=w332:string, element #2=w333:string, element #3=w335:string, element #4=w334:string)
          n166 = Array Subset "Remove\nHeader"(array=w323, index (row)=w337) -> (w322:string[][])  [unwired: 3 in]
          n167 = flat-sequence "Set Custom Step Parameters" {
            tunnel: w319 -> [w413]
            tunnel: w318 -> [w411]
            tunnel: [w410] -> w316
            frame #0 {
              w402 = bool[] [FALSE, FALSE, FALSE, FALSE, FALSE, FALSE, FALSE, FALSE]  # appended array
              n168 = Index Array "Custom Step Parameters\nSelected for Each Step"(array=w413) -> (element #1=w412:i32[], element #2=w409:i32[], element #3=w408:i32[], element #4=w407:i32[], element #5=w406:i32[], element #6=w405:i32[], element #7=w404:i32[], element #8=w403:i32[])  [unwired: 16 in]
              n169 = for {
                tunnel: w412 -> [w433] mode=indexing
                tunnel: w411 -> [w432]
                tunnel: [w431] -> w410 mode=indexing
                tunnel: w409 -> [w430] mode=indexing
                tunnel: w408 -> [w429] mode=indexing
                tunnel: w407 -> [w428] mode=indexing
                tunnel: w406 -> [w427] mode=indexing
                tunnel: w405 -> [w426] mode=indexing
                tunnel: w404 -> [w425] mode=indexing
                tunnel: w403 -> [w424] mode=indexing
                tunnel: w402 -> [w423]
                n170 = Greater Than 0?(x=w433) -> (x > 0?=w422:bool)
                n171 = Greater Than 0?(x=w430) -> (x > 0?=w421:bool)
                n172 = Greater Than 0?(x=w429) -> (x > 0?=w420:bool)
                n173 = Greater Than 0?(x=w428) -> (x > 0?=w419:bool)
                n174 = Greater Than 0?(x=w427) -> (x > 0?=w417:bool)
                n175 = Greater Than 0?(x=w426) -> (x > 0?=w416:bool)
                n176 = Greater Than 0?(x=w425) -> (x > 0?=w415:bool)
                n177 = Greater Than 0?(x=w424) -> (x > 0?=w414:bool)
                n178 = Replace Array Subset(array=w423, new element #1=w422, new element #2=w421, new element #3=w420, new element #4=w419, new element #5=w417, new element #6=w416, new element #7=w415, new element #8=w414) -> (w418:bool[])  [unwired: 8 in]
                n179 = Bundle By Name(cluster=w432, "Digital Outputs"=w418) -> (w431:cluster{"Digital Outputs":bool[]})
              }
            }
          }
          n180 = Matrix Size "Columns\nof Custom"(0:w323) -> (2:w326:i32)  [unwired: 1 out]
          n181 = To Upper Case(1:w335) -> (0:w370:string)
          n182 = Array Subset(array=w323, index (row)=w347, index (col)=w393, length (col)=w347) -> (w343:string[][])  [unwired: 1 in]
          n183 = Array Subset(array=w323, index (row)=w347, index (col)=w392, length (col)=w347) -> (w345:string[][])  [unwired: 1 in]
          n184 = Subtract(x=w326, y=w320) -> (x-y=w321:i32)
          n185 = for "Custom Step Parameters" {
            N: w321 -> [_]
            tunnel: 1 ("index") -> [w443]
            tunnel: 10 ("dimension size") -> [w442]
            tunnel: w323 -> [w441]
            tunnel: w322 -> [w440]
            tunnel: w320 -> [w438]
            tunnel: [w434] -> w319 mode=indexing
            i -> [w439]
            n186 = Add(x=w438, y=w439) -> (x+y=w437:i32)
            n187 = Array Subset(array=w441, index (row)=w443, index (col)=w437, length (col)=w443) -> (w444:string[][])  [unwired: 1 in]
            n188 = Reshape Array "Get\nOptions"(w444, w442) -> (w435:string[])
            n189 = Index Array "Select\nColumn"(array=w440, index (col)=w437) -> (element=w436:string[])  [unwired: 1 in]
            n190 = for {
              tunnel: w436 -> [w446] mode=indexing
              tunnel: w435 -> [w447]
              tunnel: [w445] -> w434 mode=indexing
              n191 = Search 1D Array "Search for\nSelection"(1D array=w447, element=w446) -> (index of element=w445:i32)  [unwired: 1 in]
            }
          }
          n192 = Reshape Array "Get\nOptions"(w343, w346) -> (w344:string[])
          n193 = Reshape Array(w345, w346) -> (w348:string[])
          n194 = Index Array "Select\nColumn"(array=w322, index (col) #1=w396, index (col) #2=w395, index (col) #3=w394, index (col) #4=w393, index (col) #5=w392) -> (element #1=w338:string[], element #2=w339:string[], element #3=w340:string[], element #4=w341:string[], element #5=w342:string[])  [unwired: 5 in]
          n195 = Equal?(x=w370, y="YES") -> (x = y?=w371:bool)
          n196 = Current VI's Path "Current\nVI's Path"() -> (path=w285:path)
          n197 = for "Standard Step Parameters" {
            tunnel: w338 -> [w462] mode=indexing
            tunnel: w339 -> [w459] mode=indexing
            tunnel: w340 -> [w457] mode=indexing
            tunnel: w341 -> [w453] mode=indexing
            tunnel: w342 -> [w449] mode=indexing
            tunnel: [w456] -> w295 mode=indexing
            tunnel: w344 -> [w454]
            tunnel: w348 -> [w450]
            n198 = Fract/Exp String To Number "String to\nNumber"(string=w462, default (0 dbl)=0) -> (number=w460:i32)  [unwired: 2 in, 1 out]
            n199 = Fract/Exp String To Number ("String to\nNumber")(string=w457) -> (number=w458:dbl)  [unwired: 3 in, 1 out]
            n200 = Search 1D Array "Search for\nSelection"(1D array=w454, element=w453) -> (index of element=w455:i32)  [unwired: 1 in]
            n201 = Search 1D Array(1D array=w450, element=w449) -> (index of element=w451:i32)  [unwired: 1 in]
            n202 = To Unsigned Word Integer(number=w451) -> (unsigned 16bit integer=w448:u16)
            n203 = To Unsigned Word Integer(number=w455) -> (unsigned 16bit integer=w452:u16)
            n204 = Bundle By Name(cluster=T6 {"Step Number"=0, "Step Description"="", "Step Time Target"=0.0, "Step Time Unit"=0, "Step End Action"=0} ("Standard Test Step Parameters"), "Step Number"=w460, "Step Description"=w459, "Step Time Target"=w458, "Step Time Unit"=w452, "Step End Action"=w448) -> (w456:T6)
          }
          n205 = Path To String(path=w285) -> (string=w290:string)
          n206 = To More Specific Class(target class=w353, reference=w362) -> (specific class reference=w349:refnum<vi>)  [unwired: 1 in, 1 out]
          n207 = To More Specific Class(target class=w367, reference=w363) -> (specific class reference=w350:refnum<vi>)  [unwired: 1 in, 1 out]
          n208 = Decimal String To Number(string=w333) -> (number=w366:i32)  [unwired: 2 in, 1 out]
          n209 = To More Specific Class(target class=w368, reference=w364) -> (specific class reference=w351:refnum<vi>)  [unwired: 1 in, 1 out]
          n210 = To More Specific Class(target class=w372, reference=w365) -> (specific class reference=w352:refnum<vi>)  [unwired: 1 in, 1 out]
          n211 = Decimal String To Number(string=w334) -> (number=w310:i32)  [unwired: 2 in, 1 out]
          n212 = Search/Split String "Find\nFile \nExtension"(string=w290, search string/char (-)=".") -> (substring before match=w289:string)  [unwired: 1 in, 2 out]
          n213 = To Variant(anything=w366) -> (Variant=w311:variant)
          n214 = To Variant(anything=w310) -> (Variant=w309:variant)
          n215 = property on="Test Description" class="Str"(reference=w349, "Value"=w332) -> ()  [unwired: 1 in, 2 out]
          n216 = property on="Loop Limit" class="DigNum"(reference=w350, "Value"=w311) -> ()  [unwired: 1 in, 2 out]
          n217 = property on="Continue at Loop Limit" class="Bool (strict)"(reference=w351, "Value"=w371) -> ()  [unwired: 1 in, 2 out]
          n218 = property on="Step N" class="DigNum"(reference=w352, "Value"=w309) -> ()  [unwired: 1 in, 2 out]
          n219 = Reverse String "Reverse"(1:w289) -> (0:w288:string)
          n220 = Search/Split String "Find\nFile \nName"(string=w288, search string/char (-)="\\") -> (match + rest of string=w286:string)  [unwired: 1 in, 2 out]
          n221 = Reverse String "Reverse"(1:w286) -> (0:w292:string)
          n222 = Unbundle By Name(w266) -> ("Max Steps"=w377:i32)
          n223 = Unbundle By Name(w266) -> ("Step Select"=w308:i32)
          n224 = Unbundle By Name(w266) -> ("New Test Name"=w301:i32)
          n225 = Unbundle By Name(w266) -> ("Test Array (Standard)"=w373:i32)
          n226 = Unbundle By Name(w266) -> ("Test Array (Custom)"=w314:i32)
          n227 = String To Path(string=w292) -> (path=w283:path)
          n228 = Empty String/Path? "Empty\nPath?"(string/path=w272) -> (empty?=w284:bool)
          n229 = Select(t=w283, s=w284, f=w272) -> (s? t:f=w293:path)
          n230 = List Folder "List Files\nin Folder"(path=w293, pattern="*.txt", error in=w275) -> (filenames=w264:string[], error out=w274:errorcluster)  [unwired: 3 out]
          n231 = Index Array(array=w265, index=w301) -> (element=w300:refnum<vi>)
          n232 = Index Array(array=w265, index=w377) -> (element=w329:refnum<vi>)
          n233 = Index Array(array=w265, index=w308) -> (element=w304:refnum<vi>)
          n234 = Index Array(array=w265, index=w373) -> (element=w374:refnum<vi>)
          n235 = Index Array(array=w265, index=w314) -> (element=w313:refnum<vi>)
          n236 = for "Remove Extension" {
            tunnel: w264 -> [w400] mode=indexing
            tunnel: ".txt" ("pattern") -> [w401]
            tunnel: [w399] -> w276 mode=indexing
            tunnel: [w398] -> w281 mode=indexing
            n237 = Search and Replace String(input string=w400, search string=w401) -> (result string=w399:string, number of replacements=w398:i32)  [unwired: 6 in, 2 out]
          }
          n238 = To More Specific Class(target class=w302, reference=w300) -> (specific class reference=w299:refnum<vi>)  [unwired: 1 in, 1 out]
          n239 = To More Specific Class(target class=refnum<vi> refnum ("Max Steps"), reference=w329) -> (specific class reference=w331:refnum<vi>)  [unwired: 1 in, 1 out]
          n240 = To More Specific Class(target class=w307, reference=w304) -> (specific class reference=w305:refnum<vi>)  [unwired: 1 in, 1 out]
          n241 = To More Specific Class(target class=w375, reference=w374) -> (specific class reference=w376:refnum<vi>)  [unwired: 1 in, 1 out]
          n242 = To More Specific Class(target class=w312, reference=w313) -> (specific class reference=w315:refnum<vi>)  [unwired: 1 in, 1 out]
          n243 = Array Size(array=w295) -> (size(s)=w327:i32)
          n244 = Add Array Elements(numeric array=w281) -> (sum=w280:i32)
          n245 = Equal To 0?(x=w280) -> (x = 0?=w279:bool)
          n246 = To Variant(anything=w327) -> (Variant=w328:variant)
          n247 = To Variant(anything=u32 0) -> (Variant=w306:variant)
          n248 = Build Array(u32 0) -> (w296:u32[])
          n249 = To Variant(anything=w316) -> (Variant=w317:variant)
          n250 = Select(t=string[] ["No Tests Found"], s=w279, f=w276) -> (s? t:f=w278:string[])
          n251 = property on="Loop Limit" class="Str"(reference=w299, "Visible"=FALSE, "Value"=w298) -> ()  [unwired: 1 in, 2 out]
          n252 = property on="Test Array (Custom)" class="Arr"(reference=w315, "Value"=w317, "Index Values"=w296) -> ()  [unwired: 1 in, 2 out]
          n253 = property on="Max Steps" class="DigNum"(reference=w331, "Value"=w328) -> ()  [unwired: 1 in, 2 out]
          n254 = property on="Step Select" class="DigNum"(reference=w305, "Value"=w306) -> ()  [unwired: 1 in, 2 out]
          n255 = property on="Test Array (Standard)" class="Arr (strict)"(reference=w376, "Value"=w295, "Index Values"=w296) -> ()  [unwired: 1 in, 2 out]
          n256 = property on="Set\nAvailable Tests" class="Ring"(reference=w270, "Strings []"=w278) -> ()  [unwired: 1 in, 2 out]
        }
      }
    }
    frame True {
      # "Alternating\nBoolean State\n(Starts @ FALSE)"
      n257 = First Call?() -> (First Call?: T/F=w474:bool)
      n258 = feedback #7(w474) -> (w475:bool)
      n259 = Not(x=w475) -> (.not. x?=w473:bool)
      n260 = feedback-in #7(w473) -> ()
      n261 = case "Save Test?" shown="True" w473 {
        tunnel: w471 -> [_ w507]
        tunnel: w472 -> [_ w508]
        tunnel: w470 -> [w483 w537]
        tunnel: w469 -> [w480 w541]
        tunnel: w468 -> [w479 w536]
        tunnel: w467 -> [_ w500]
        tunnel: w466 -> [_ w499]
        tunnel: w465 -> [_ w512]
        tunnel: [w476 w513] -> w464
        frame False {
          w476 = errorcluster {"status"=FALSE, "code"=0, "source"=""}  # No Error
          w485 = ""  # Empty
          # "2nd Disable Save Button until New Test Name is valid"
          # "1st   New Test Name : Clear, Enable, Visible."
          n262 = To Variant(anything=FALSE ("Value")) -> (Variant=w481:variant)
          n263 = One Button Dialog(message="Please Enter A New Test Name and Click Save Test Again.") -> ()  [unwired: 1 in, 1 out]
          n264 = property on="Save Test" class="Bool"(reference=w483, "Value"=w481, "DisabledEnum"=T3."Disabled and Grayed Out" ("Disabled")) -> ()  [unwired: 1 in, 2 out]
          n265 = property on="New Test Name" class="Str"(reference=w480, "Value"=w485, "DisabledEnum"=T3."Enabled" ("Disabled"), "Visible"=TRUE) -> ()  [unwired: 1 in, 2 out]
          n266 = property on="Load Test" class="Ring"(reference=w479, "DisabledEnum"=T3."Disabled and Grayed Out" ("Disabled")) -> ()  [unwired: 1 in, 2 out]
        }
        frame True {
          w493 = string[] [" ", "", "", "", " "]  # Blank Standard Row
          w495 = errorcluster {"status"=FALSE, "code"=0, "source"=""}  # No Error
          w502 = 5  # Cols in Standard Template
          w504 = 1  # Option Start Index
          w503 = 10  # Max Num Options
          w509 = refnum<vi> refnum  # Test Array (Custom)
          w550 = refnum<vi> refnum  # Digital
          w568 = refnum<vi> refnum  # Boolean
          w559 = 12  # Sequence Start Index (Row)
          w579 = string[] ["sec", "min", "hr"]  # Step Time Units (Text)
          w578 = string[] ["Go to Next Step", "Loop to Step 0", "Loop to Step N", "Stop Test Mode", "Stop Program"]  # Step End Actions (Text)
          w580 = refnum<vi> refnum  # Test Array (Standard)
          w596 = refnum<vi> refnum  # String
          w604 = 6  # Step N Index (Row)
          w607 = 5  # Continue at Loop Limit Index (Row)
          w605 = 4  # Loop Limit Index (Row)
          w606 = 3  # Test Description Index (Row)
          w603 = 1  # Details Index (Col)
          # "Convert Custom Parameters\nto\nOption Index Values"
          # "Convert Option Index Values\nto\nCustom Test String Values"
          # "Write Test Sequence\nTo Text File"
          # "Convert Test Sequence Details into Strings"
          # "Convert Test Sequence Parameters\ninto String Array \"New Test Values\""
          n267 = property on="New Test Name" class="Str"(reference=w541) -> (reference out=w540:refnum<vi>, "Value"=w542:string)  [unwired: 1 in, 1 out]
          n268 = Unbundle By Name(w507) -> ("Test Description"=w591:i32, "Loop Limit"=w594:i32, "Continue at Loop Limit"=w593:i32, "Step N"=w592:i32)
          n269 = Unbundle By Name(w507) -> ("Test Array (Custom)"=w510:i32)
          n270 = Unbundle By Name(w507) -> ("Test Array (Standard)"=w583:i32)
          n271 = Current VI's Path "Current\nVI's Path"() -> (path=w525:path)
          n272 = Path To String(path=w512) -> (string=w569:string)
          n273 = Path To String(path=w525) -> (string=w530:string)
          n274 = Concatenate Strings(w569, "\\" ("string"), w542, ".txt" ("string")) -> (w588:string)
          n275 = Search/Split String "Find\nFile \nExtension"(string=w530, search string/char (-)=".") -> (substring before match=w529:string)  [unwired: 1 in, 2 out]
          n276 = String To Path(string=w588) -> (path=w584:path)
          n277 = Index Array(array=w508, index=w510) -> (element=w506:refnum<vi>)
          n278 = Reverse String "Reverse"(1:w529) -> (0:w528:string)
          n279 = Index Array(array=w508, index #1=w591, index #2=w594, index #3=w593, index #4=w592) -> (element #1=w602:refnum<vi>, element #2=w599:refnum<vi>, element #3=w567:refnum<vi>, element #4=w595:refnum<vi>)
          n280 = To Variant(anything=FALSE ("Value")) -> (Variant=w538:variant)
          n281 = Index Array(array=w508, index=w583) -> (element=w582:refnum<vi>)
          n282 = Array Subset "Parameter\nOptions"(array=w500, index (row)=w504, length (row)=w503, index (col)=w502) -> (w489:string[][])  [unwired: 1 in]
          n283 = To More Specific Class(target class=w509, reference=w506) -> (specific class reference=w505:refnum<vi>)  [unwired: 1 in, 1 out]
          n284 = property on="Save Test" class="Bool"(reference=w537, "Value"=w538) -> ()  [unwired: 1 in, 2 out]
          n285 = To More Specific Class(target class=w580, reference=w582) -> (specific class reference=w581:refnum<vi>)  [unwired: 1 in, 1 out]
          n286 = Open/Create/Replace File(file path (use dialog)=w584, error in=w495, operation (0:open)=T5."replace or create") -> (refnum out=w585:refnum<file>, error out=w587:errorcluster)  [unwired: 3 in, 1 out]
          n287 = Search/Split String "Find\nFile \nName"(string=w528, search string/char (-)="\\") -> (match + rest of string=w526:string)  [unwired: 1 in, 2 out]
          n288 = To More Specific Class(target class=w596, reference=w602) -> (specific class reference=w601:refnum<vi>)  [unwired: 1 in, 1 out]
          n289 = property class="Arr"(reference=w505) -> ("Value"=w498:variant)  [unwired: 1 in, 2 out]
          n290 = To More Specific Class(target class=w550, reference=w599) -> (specific class reference=w598:refnum<vi>)  [unwired: 1 in, 1 out]
          n291 = property class="Arr (strict)"(reference=w581) -> ("Value"=w494:T4)  [unwired: 1 in, 2 out]
          n292 = Read from Text File(file (use dialog)=w585, error in=w587) -> (refnum out=w571:refnum<file>, error out=w570:errorcluster)  [unwired: 4 out]
          n293 = Reverse String "Reverse"(1:w526) -> (0:w532:string)
          n294 = To More Specific Class(target class=w568, reference=w567) -> (specific class reference=w546:refnum<vi>)  [unwired: 1 in, 1 out]
          n295 = To More Specific Class(target class=w550, reference=w595) -> (specific class reference=w597:refnum<vi>)  [unwired: 1 in, 1 out]
          n296 = String To Path(string=w532) -> (path=w523:path)
          n297 = Variant To Data(type=w499, Variant=w498) -> (data=w492:cluster{"Digital Outputs":bool[]}[])  [unwired: 1 in, 1 out]
          n298 = property class="Str"(reference=w601) -> ("Value"=w600:string)  [unwired: 1 in, 2 out]
          n299 = property class="DigNum"(reference=w598) -> ("Value"=w552:variant)  [unwired: 1 in, 2 out]
          n300 = property class="Bool"(reference=w546) -> ("Value"=w545:variant)  [unwired: 1 in, 2 out]
          n301 = property class="DigNum"(reference=w597) -> ("Value"=w549:variant)  [unwired: 1 in, 2 out]
          n302 = for {
            tunnel: w494 -> [w653] mode=indexing
            tunnel: w579 -> [w648]
            tunnel: w578 -> [w647]
            tunnel: [w639] -> w496 mode=indexing
            tunnel: w493 -> [w636]
            n303 = Unbundle By Name(w653) -> ("Step Number"=w643:i32, "Step Description"=w641:string, "Step Time Target"=w649:dbl, "Step Time Unit"=w646:u16, "Step End Action"=w645:u16)
            n304 = To Long Integer(number=w646) -> (32bit integer=w651:i32)
            n305 = To Long Integer(number=w645) -> (32bit integer=w652:i32)
            n306 = Number To Fractional String(number=w643, precision (6)=i16 0) -> (F-format string=w642:string)  [unwired: 2 in]
            n307 = Number To Fractional String(number=w649, precision (6)=i16 3) -> (F-format string=w640:string)  [unwired: 2 in]
            n308 = Index Array(array=w648, index=w651) -> (element=w638:string)
            n309 = Index Array(array=w647, index=w652) -> (element=w637:string)
            n310 = Replace Array Subset "Insert\nValues"(array=w636, new element #1=w642, new element #2=w641, new element #3=w640, new element #4=w638, new element #5=w637) -> (w639:string[])  [unwired: 5 in]
          }
          n311 = Empty String/Path? "Empty\nPath?"(string/path=w512) -> (empty?=w524:bool)
          n312 = Variant To Data(type=u16 0, Variant=w552) -> (data=w551:u16)  [unwired: 1 in, 1 out]
          n313 = Variant To Data(type=FALSE, Variant=w545) -> (data=w543:bool)  [unwired: 1 in, 1 out]
          n314 = Variant To Data(type=u16 0, Variant=w549) -> (data=w547:u16)  [unwired: 1 in, 1 out]
          n315 = Select "Use Default\nLocation?"(t=w523, s=w524, f=w512) -> (s? t:f=w533:path)
          n316 = Number To Fractional String(number=w547, precision (6)=i16 0) -> (F-format string=w560:string)  [unwired: 2 in]
          n317 = Number To Fractional String(number=w551, precision (6)=i16 0) -> (F-format string=w562:string)  [unwired: 2 in]
          n318 = Select(t="YES", s=w543, f="NO") -> (s? t:f=w564:string)
          n319 = Replace Array Subset "Update\nTest Detail\nCells"(array=w500, new element #1=w600, index (row) #1=w606, index (col) #1=w603, new element #2=w562, index (row) #2=w605, index (col) #2=w603, new element #3=w564, index (row) #3=w607, index (col) #3=w603, new element #4=w560, index (row) #4=w604, index (col) #4=w603) -> (w558:string[][])
          n320 = property on="New Test Name" class="Str"(reference=w540, "Visible"=FALSE) -> ()  [unwired: 1 in, 2 out]
          n321 = Array Subset "Details\nOnly"(array=w558, length (row)=w559) -> (w557:string[][])  [unwired: 3 in]
          n322 = Matrix Size(0:w489) -> (2:w490:i32)  [unwired: 1 out]
          n323 = Initialize Array "Blank\nCustom Row (Indexes)"(0 ("32bit integer"), w490) -> (w488:i32[])
          n324 = for "Index by Test Steps" {
            tunnel: [w615] -> w501 mode=indexing
            tunnel: w492 -> [w618] mode=indexing
            tunnel: w488 -> [w617]
            n325 = Unbundle By Name(w618) -> ("Digital Outputs"=w620:bool[])
            n326 = Boolean To (0,1)(Boolean=w620) -> (0, 1=w619:i16[])
            n327 = To Long Integer(number=w619) -> (32bit integer=w616:i32[])
            n328 = Replace Array Subset "Insert\nValues"(array=w617, new element=w616) -> (w615:i32[])  [unwired: 1 in]
          }
          n329 = for "Index Test Steps" {
            tunnel: w501 -> [w610] mode=indexing
            tunnel: w489 -> [w609]
            tunnel: [w608] -> w497 mode=indexing
            n330 = for "Index Parameters" {
              tunnel: w610 -> [w614] mode=indexing
              tunnel: w609 -> [w611]
              tunnel: [w613] -> w608 mode=indexing
              i -> [w612]
              n331 = Index Array "Select\nOption"(array=w611, index (row)=w614, index (col)=w612) -> (element=w613:string)
            }
          }
          n332 = Insert Into Array "Combine\nStandard\nand Custom\nTest Values"(array=w496, index (col)=5 ("disabled index (col)"), new element=w497) -> (w556:string[][])  [unwired: 1 in]
          n333 = Insert Into Array "Combine\nDetails and\nNew Test Values"(array=w557, new element=w556) -> (w555:string[][])  [unwired: 2 in]
          n334 = Array To Spreadsheet String "Array To \nSpreadsheet String"(delimiter (Tab)="\t" ("delimiter (\\t)"), array=w555, 3:"%s" ("format (%s)")) -> (spreadsheet string=w574:string)
          n335 = Write to Text File ("Write to\nText File")(file (use dialog)=w571, text=w574, error in=w570) -> (refnum out=w573:refnum<file>, error out=w572:errorcluster)  [unwired: 1 in, 1 out]
          n336 = Close File(refnum=w573, error in=w572) -> (error out=w553:errorcluster)  [unwired: 1 out]
          n337 = case shown="No Error" w553 {
            selector: w553 -> [w626 w635]
            tunnel: w569 -> [w634 _]
            tunnel: w542 -> [w627 _]
            tunnel: [w626 w635] -> w515
            frame No Error {
              w632 = "\r\n"
              w630 = "\""
              n338 = Concatenate Strings(w632, w632) -> (w628:string)
              n339 = Concatenate Strings("Test Sequence:", w628, w630, w627, w630, w628, "Was Saved Successfully to the Test Folder:", w628, w634, w628) -> (w633:string)
              n340 = One Button Dialog "Display\nSave Info"(message=w633) -> ()  [unwired: 1 in, 1 out]
            }
            frame Error {
            }
          }
          n341 = List Folder "List Files\nin Folder"(path=w533, pattern="*.txt", error in=w515) -> (filenames=w535:string[], error out=w513:errorcluster)  [unwired: 3 out]
          n342 = for "Remove Extension" {
            tunnel: w535 -> [w624] mode=indexing
            tunnel: ".txt" ("pattern") -> [w625]
            tunnel: [w623] -> w516 mode=indexing
            tunnel: [w621] -> w521 mode=indexing
            n343 = Search and Replace String(replace all?=TRUE ("replace all? (F)"), input string=w624, search string=w625) -> (result string=w623:string, number of replacements=w621:i32)  [unwired: 5 in, 2 out]
          }
          n344 = Add Array Elements(numeric array=w521) -> (sum=w520:i32)
          n345 = Equal To 0?(x=w520) -> (x = 0?=w519:bool)
          n346 = Select(t=string[] ["No Tests Found"], s=w519, f=w516) -> (s? t:f=w518:string[])
          n347 = property on="Load Test Ring" class="Ring"(reference=w536, "DisabledEnum"=T3."Enabled" ("Disabled"), "Strings []"=w518) -> ()  [unwired: 1 in, 2 out]
        }
      }
    }
  }
  n348 = case shown="No Error" w10 {
    selector: w10 -> [_ w869]
    tunnel: w9 -> [w658 _]
    tunnel: [errorcluster {"status"=FALSE, "code"=0, "source"=""} ("error IO") w869] -> w33
    tunnel: w22 -> [w671 _]
    tunnel: w23 -> [w670 _]
    tunnel: w24 -> [w669 _]
    tunnel: "NEXT STEP" -> [w668 _]
    tunnel: "HOLD STEP" -> [w667 _]
    tunnel: string[][] [[" seconds", "1"], [" minutes", "60"], [" hours", "3600"]] ("appended array") -> [w666 _]
    tunnel: "START TEST" -> [w657 _]
    tunnel: "STOP TEST" -> [w665 _]
    tunnel: [w664 w868] -> w12
    tunnel: [w663 w867] -> w17
    tunnel: [w662 w867] -> w16
    tunnel: [w661 w866] -> w15
    tunnel: [w660 w866] -> w14
    tunnel: [w659 "TEST ERROR"] -> w13
    frame No Error {
      w675 = "\r"
      # "Test Display:\nMode:\nStep Description:\nStep Time:\nStep 1 of 100   Loop 1 of 100"
      # "Step End Actions:\n0:  Go to Next Step\n1:  Loop to Step 0\n2:  Loop to Step N\n3:  Stop Test Mode\n4:  Stop Program"
      n349 = Array Size(array=w658) -> (size(s)=w654:i32)
      n350 = Greater Than 0?(x=w654) -> (x > 0?=w656:bool)
      n351 = And(x=w657, y=w656) -> (x .and. y?=w655:bool)
      n352 = First Call? "First\nCall?"() -> (First Call?: T/F=w676:bool)
      n353 = for {
        N: 1 -> [_]
        tunnel: w668 -> [w700]
        tunnel: [w724] -> w683
        tunnel: w665 -> [w702]
        tunnel: w667 -> [w696]
        tunnel: [w726] -> w680
        tunnel: [w725] -> w678
        tunnel: [w722] -> w684
        tunnel: [w718] -> w681
        shift-right: [w720] -> w663
        shift-left: _ -> [w711]
        shift-right: [w719] -> w662
        shift-left: _ -> [w717]
        shift-right: [w721] -> w660
        shift-left: _ -> [w698]
        tunnel: w669 -> [w716]
        tunnel: w670 -> [w715]
        tunnel: w671 -> [w714]
        tunnel: w658 -> [w709]
        tunnel: w666 -> [w712]
        tunnel: [w723] -> w674
        shift-right: [w706] -> _
        shift-left: _ -> [w694]
        tunnel: [w705] -> w664
        tunnel: w676 -> [w695]
        tunnel: u16 0 ("t") -> [w704]
        tunnel: w655 -> [w692]
        tunnel: w654 -> [w691]
        n354 = Select(t=w704, s=w695, f=w711) -> (s? t:f=w708:u16)
        n355 = Select(t=w704, s=w695, f=w717) -> (s? t:f=w713:u16)
        n356 = feedback-in #8(w700) -> ()
        n357 = feedback #8() -> (w701:bool)  [unwired: 1 in]
        n358 = To Long Integer(number=w708) -> (32bit integer=w710:i32)
        n359 = To Unsigned Word Integer(number=w691) -> (unsigned 16bit integer=w693:u16)
        n360 = Greater? "Pulse on\nTRUE"(x=w700, y=w701) -> (0:w699:bool)
        n361 = Index Array "Index\nTest Array"(array=w709, index=w710) -> (element=w707:T6)
        n362 = Compound Arithmetic op=OR "Stop\nTest?"(w702, w694, w695) -> (w703:bool)
        n363 = while "Boolean Latch Function" {
          tunnel: w692 -> [w731]
          shift-right: [w729] -> w705
          shift-left: _ -> [w730]
          tunnel: w703 -> [w727]
          stop <- FALSE continue-if-true
          n364 = Exclusive Or(1:w727, 2:w731) -> (0:w732:bool)
          n365 = Select(t=w731, s=w732, f=w730) -> (s? t:f=w729:bool)
        }
        n366 = Compound Arithmetic op=OR "Reset\nTimer?"(w695, w698, w696) -> (w697:bool)
        n367 = case "Test Running?" shown="True" w705 {
          tunnel: ["Mode: OFF  (Press Start to Begin)" w804] -> w718
          tunnel: w708 -> [_ w742]
          tunnel: [w735 w805] -> w723
          tunnel: w696 -> [_ w773]
          tunnel: [w738 w807] -> w720
          tunnel: [w736 w751] -> w721
          tunnel: [w737 w806] -> w719
          tunnel: w713 -> [_ w741]
          tunnel: w714 -> [_ w755]
          tunnel: [w733 w801] -> w726
          tunnel: [w733 w776] -> w725
          tunnel: [w733 w799] -> w722
          tunnel: [w733 w782] -> w724
          tunnel: w699 -> [_ w774]
          tunnel: w715 -> [_ w798]
          tunnel: w712 -> [_ w797]
          tunnel: w716 -> [_ w754]
          tunnel: w693 -> [_ w757]
          tunnel: w707 -> [_ w750]
          tunnel: [w734 w783] -> w706
          tunnel: w697 -> [_ w763]
          frame False {
            w734 = FALSE  # Stop Test Mode
            w733 = ""  # Empty
            w735 = FALSE  # Stop Program
            w736 = TRUE  # Step Complete Signal
            w737 = u16 0  # Loop Count
            w738 = u16 0  # Test Step
          }
          frame True {
            w745 = " / " ("string")
            w778 = ""  # Empty
            w786 = ""  # Empty
            w759 = i16 1 ("width (-)")
            n368 = Decrement "Last Step"(x=w757) -> (x-1=w752:u16)
            n369 = Number To Fractional String(number=w741, precision (6)=i16 0 ("width (-)")) -> (F-format string=w740:string)  [unwired: 2 out]
            n370 = Unbundle By Name(w750) -> ("Step Description"=w782:string)
            n371 = Unbundle By Name(w750) -> ("Step Time Unit"=w761:u16, "Step Time Target"=w760:dbl)
            n372 = Unbundle By Name(w750) -> ("Step End Action"=w753:u16)
            n373 = Tick Count (ms)() -> (millisecond timer value=w769:u32)
            n374 = Number To Fractional String(number=w742, precision (6)=i16 0 ("width (-)")) -> (F-format string=w743:string)  [unwired: 2 out]
            n375 = feedback #9() -> (w771:u32)  [unwired: 1 in]
            n376 = feedback #10() -> (w768:u32)  [unwired: 1 in]
            n377 = feedback-in #10(w769) -> ()
            n378 = To Long Integer(number=w761) -> (32bit integer=w792:i32)
            n379 = Index Array(array=w797, index (row) #1=w792, index (col) #1=0 ("disabled index (col)"), index (row) #2=w792, index (col) #2=1 ("index (col)")) -> (element #1=w747:string, element #2=w790:string)
            n380 = Subtract(x=w769, y=w768) -> (x-y=w764:u32)
            n381 = Add(x=w771, y=w764) -> (x+y=w772:u32)
            n382 = Select "Reset\nTimer?"(t=u32 0 ("x+y"), s=w763, f=w772) -> (s? t:f=w770:u32)
            n383 = feedback-in #9(w770) -> ()
            n384 = To Double Precision Float(number=w770) -> (double precision float=w765:dbl)
            n385 = Divide "Elapsed\nTime [s]"(x=w765, y=1000.0) -> (x/y=w762:dbl)
            n386 = Fract/Exp String To Number "Get Unit\nMultiplier"(string=w790) -> (number=w789:dbl)  [unwired: 3 in, 1 out]
            n387 = Divide(x=w762, y=w789) -> (x/y=w791:dbl)
            n388 = Multiply "Time Target\n(seconds)"(x=w760, y=w789) -> (x*y=w784:dbl)
            n389 = Number To Fractional String(number=w752, precision (6)=i16 0 ("width (-)")) -> (F-format string=w756:string)  [unwired: 2 out]
            n390 = Number To Fractional String(number=w755, precision (6)=i16 0 ("width (-)")) -> (F-format string=w744:string)  [unwired: 2 out]
            n391 = Greater Or Equal? "Step Time\nElapsed?"(x=w762, y=w784) -> (x >= y?=w758:bool)
            n392 = Or "Step\nComplete?"(x=w758, y=w774) -> (x .or. y?=w751:bool)
            n393 = case shown="True" w751 {
              tunnel: [w811 w822] -> w807
              tunnel: [w810 w821] -> w806
              tunnel: [w809 w820] -> w805
              tunnel: w798 -> [_ w819]
              tunnel: w741 -> [w810 w818]
              tunnel: [w808 w817] -> w783
              tunnel: w742 -> [w811 w816]
              tunnel: w753 -> [_ w815]
              tunnel: w755 -> [_ w814]
              tunnel: w754 -> [_ w813]
              tunnel: w752 -> [_ w812]
              frame False {
                w809 = FALSE  # Stop Program
                w808 = FALSE  # Stop Test Mode
                # "Continue With Current Step"
              }
              frame True {
                n394 = case "Step End Actions" shown="1" w815 {
                  tunnel: [w827 w836 w851 w860 w863] -> w822
                  tunnel: [w826 w842 w856 w857 w864] -> w820
                  tunnel: [w828 w829 w846 w858 w861] -> w821
                  tunnel: w816 -> [w825 w838 w852 _ _]
                  tunnel: w818 -> [w828 w830 w845 w858 w861]
                  tunnel: [w823 w839 w853 w859 w862] -> w817
                  tunnel: w819 -> [_ _ w843 _ _]
                  tunnel: w814 -> [_ w841 w855 _ _]
                  tunnel: w813 -> [_ w834 w849 _ _]
                  tunnel: w812 -> [w824 _ _ _ _]
                  frame 0, Default {
                    w826 = FALSE  # Stop Program
                    # "Continue to Next\nTest Step"
                    n395 = Equal? "Last\nStep?"(x=w825, y=w824) -> (x = y?=w823:bool)
                    n396 = Increment(x=w825) -> (x+1=w827:u16)
                  }
                  frame 1 {
                    w840 = FALSE  # Stop Test?
                    w842 = FALSE  # Stop Program
                    w837 = u16 0  # Step #
                    # "Loop to\nTest Step 0"
                    n397 = Greater Or Equal? "Loop\nLimit?"(x=w830, y=w841) -> (x >= y?=w833:bool)
                    n398 = Increment(x=w838) -> (x+1=w835:u16)
                    n399 = Increment(x=w830) -> (x+1=w831:u16)
                    n400 = And(x=w834, y=w833) -> (x .and. y?=w832:bool)
                    n401 = Select(t=w840, s=w834, f=w833) -> (s? t:f=w839:bool)
                    n402 = Select "Next Step?"(t=w835, s=w832, f=w837) -> (s? t:f=w836:u16)
                    n403 = Select(t=w830, s=w832, f=w831) -> (s? t:f=w829:u16)
                  }
                  frame 2 {
                    w854 = FALSE  # Stop Test?
                    w856 = FALSE  # Stop Program
                    # "Loop to\nTest Step N"
                    n404 = Greater Or Equal? "Loop\nLimit?"(x=w845, y=w855) -> (x >= y?=w848:bool)
                    n405 = Increment(x=w852) -> (x+1=w850:u16)
                    n406 = Increment(x=w845) -> (x+1=w847:u16)
                    n407 = And(x=w849, y=w848) -> (x .and. y?=w844:bool)
                    n408 = Select(t=w854, s=w849, f=w848) -> (s? t:f=w853:bool)
                    n409 = Select "Next Step?"(t=w850, s=w844, f=w843) -> (s? t:f=w851:u16)
                    n410 = Select(t=w845, s=w844, f=w847) -> (s? t:f=w846:u16)
                  }
                  frame 3 {
                    w857 = FALSE  # Stop Program
                    w859 = TRUE  # Stop Test Mode
                    w860 = u16 0  # Step #
                    # "De-Activate \nTest Mode"
                  }
                  frame 4 {
                    w862 = FALSE  # Stop Test Mode
                    w863 = u16 0  # Step #
                    w864 = TRUE  # Stop Program
                    # "Stop Entire\nLabVIEW Program"
                  }
                }
              }
            }
            n411 = Equal To 0? "No Loops?"(x=w755) -> (x = 0?=w775:bool)
            n412 = Number To Fractional String "Time\nTarget"(number=w760, precision (6)=w759) -> (F-format string=w748:string)  [unwired: 2 out]
            n413 = Number To Fractional String "Time \nElapsed"(number=w791, precision (6)=w759) -> (F-format string=w795:string)  [unwired: 2 out]
            n414 = Concatenate Strings("Step: ", w743, w745, w756) -> (w801:string)
            n415 = Concatenate Strings("Loop: ", w740, w745, w744) -> (w777:string)
            n416 = Concatenate Strings("Time: ", w795, " of ", w748, w747, "." ("string")) -> (w785:string)
            n417 = Select "Hide\nLoop Text?"(t=w778, s=w775, f=w777) -> (s? t:f=w776:string)
            n418 = Select "Hold\nStep?"(t="Mode: HOLD", s=w773, f="Mode: RUN") -> (s? t:f=w804:string)
            n419 = Select(t=w786, s=w773, f=w785) -> (s? t:f=w799:string)
          }
        }
      }
      n420 = First Call?() -> (First Call?: T/F=w673:bool)
      n421 = while "Boolean Latch Function" {
        tunnel: w674 -> [w689]
        shift-right: [w687] -> w661
        shift-left: _ -> [w688]
        tunnel: w673 -> [w685]
        stop <- FALSE continue-if-true
        n422 = Exclusive Or(1:w685, 2:w689) -> (0:w690:bool)
        n423 = Select(t=w689, s=w690, f=w688) -> (s? t:f=w687:bool)
      }
      n424 = Concatenate Strings(w681, w675, w683, w675, w684, w675, w680, "    " ("String"), w678) -> (w659:string)
    }
    frame Error {
      w866 = FALSE ("Stop Program")
      w867 = u16 0 ("Step #")
      w868 = FALSE  # Test Not Active if Error Present
    }
  }
  "Error Output" <- w33
  "Step Number" <- w17
  "Loop Number" <- w16
  "Stop Program?" <- w15
  "Step Complete?" <- w14
  "Test Display" <- w13
  "Test Running?" <- w12
  n425 = feedback-in #1(w12) -> ()
  n426 = Exclusive Or "State Change?"(1:w28, 2:w12) -> (0:w27:bool)
  n427 = Or(x=w27, y=w25) -> (x .or. y?=w26:bool)
  n428 = case "Disable Controls when Test is Running" shown="True" w26 {
    tunnel: w64 -> [_ w888]
    tunnel: w12 -> [_ w870]
    tunnel: w63 -> [_ w883]
    tunnel: w25 -> [_ w872]
    frame False {
    }
    frame True {
      n429 = Unbundle By Name(w888) -> ("Save Test"=w887:i32, "Erase Test"=w886:i32, "Test Description"=w882:i32, "Load Test Ring"=w881:i32, "Test Array (Standard)"=w880:i32, "Test Array (Custom)"=w879:i32)
      n430 = Select(t=FALSE, s=w872, f=w870) -> (s? t:f=w871:bool)
      n431 = Select(t=T3."Disabled" ("Disabled"), s=w871, f=T3."Enabled" ("Disabled")) -> (s? t:f=w874:T3)
      n432 = Index Array(array=w883, index #1=w887, index #2=w886, index #3=w882, index #4=w881, index #5=w880, index #6=w879) -> (element #1=w885:refnum<vi>, element #2=w884:refnum<vi>, element #3=w878:refnum<vi>, element #4=w877:refnum<vi>, element #5=w876:refnum<vi>, element #6=w875:refnum<vi>)
      n433 = property class="Ctl"(reference=w885, "DisabledEnum"=w874) -> ()  [unwired: 1 in, 2 out]
      n434 = property class="Ctl"(reference=w884, "DisabledEnum"=w874) -> ()  [unwired: 1 in, 2 out]
      n435 = property class="Ctl"(reference=w878, "DisabledEnum"=w874) -> ()  [unwired: 1 in, 2 out]
      n436 = property class="Ctl"(reference=w877, "DisabledEnum"=w874) -> ()  [unwired: 1 in, 2 out]
      n437 = property class="Ctl"(reference=w876, "DisabledEnum"=w874) -> ()  [unwired: 1 in, 2 out]
      n438 = property class="Ctl"(reference=w875, "DisabledEnum"=w874) -> ()  [unwired: 1 in, 2 out]
    }
  }
  n439 = Unbundle By Name("SLAM Test Cluster") -> ("Test Array (Custom)"=w4:cluster{"Digital Outputs":bool[]}[])
  n440 = To Long Integer(number=w17) -> (32bit integer=w18:i32)
  n441 = Index Array "Index Custom Array"(array=w4, index=w18) -> (element=w3:cluster{"Digital Outputs":bool[]})
  n442 = Select "Test\nRunning?"(t=w3, s=w12, f=w2) -> (s? t:f=→"Test Output":cluster{"Digital Outputs":bool[]})
